vi "Measurement Logic.vi"() -> ()   [LabVIEW 2021, in "Arbitrary Mode_PMIC.lvlib"]
uses:
  Arbitrary Mode_PMIC.lvlib
  <vilib>/Plug-In SDKs/Measurements/Measure Call Context/Measure Call Context.lvclass
  Measurement Results.ctl
  Measurement Configuration.ctl
  <instrlib>/niDCPower/nidcpower.llb/niDCPower Source Mode.ctl
  <instrlib>/niDCPower/nidcpower.llb/niDCPower Wait For Event - Event.ctl
  <instrlib>/niScope/Controls/niScope trigger slope.ctl
  <instrlib>/niDCPower/nidcpower.llb/niDCPower Output Function.ctl
  <instrlib>/niDCPower/nidcpower.llb/niDCPower Aperture Time Units.ctl
  <instrlib>/niDCPower/nidcpower.llb/niDCPower Get Channel Name From String.vi
  <instrlib>/niScope/Utility/niScope Get Channel Name From String.vi
  <instrlib>/niScope/Configure/Trigger/niScope Configure Trigger Digital.vi
  <instrlib>/niDCPower/nidcpower.llb/niDCPower Configure Digital Edge Measure Trigger With Channels.vi
  <instrlib>/niDCPower/nidcpower.llb/niDCPower Configure Digital Edge Source Trigger With Channels.vi
  <instrlib>/niScope/Acquire/Fetch/niScope Fetch WDT.vi
panel:
  in  "measurement configuration":T1={"Source maximum power"=300.0, "Source sample rate"=1800000.0, "Source current limit"=0.25, "Source resource name"="", "Source voltage pole-zero ratio"=2.0, "Source voltage compensation frequency"=3530.0, "Source voltage gain bandwidth"=2000.0, "Source transient response"=1042, "Source set-up voltage"=0.0, "Trapezoid signal enable/disable"=TRUE, "Trapezoid voltage delay t2"=0.005, "Trapezoid voltage delay t1"=0.005, "Trapezoid voltatge pulse duration"=0.005, "Trapezoid voltage rising slew rate"=24.0, "Trapezoid voltage falling slew rate"=24.0, "Trapezoid voltage set point 2(V2)"=20.0, "Trapezoid voltage set point 1(V1)"=7.0, "Ramp signal enable/disable"=FALSE, "Ramp voltage V1 time"=0.005, "Ramp voltatge V2 time"=0.005, "Ramp voltage ramp rate"=6550.0, "Ramp voltage set point 2(V2)"=20.0, "Ramp voltage set point 1(V1)"=7.0, "Source signal logging"=[], "Source signal loop count"=1, "Source sense"=1009, "Load enable/disable"=FALSE, "Load resource name"="", "Load sense"=1009, "Load voltage limit range"=4.0, "Load current level range"=4.0, "Load current level"=0.03, "Load transient response"=1042, "Load current gain bandwidth"=14000.0, "Load current compensation frequency"=180000.0, "Load current pole-zero ratio"=0.3, "Scope enable/disable"=FALSE, "Scope resource name"="", "Scope output channel name"="0", "Scope sample rate"=1800000.0, "Scope probe attenuation"=1.0, "Scope vertical range"=10.0, "Scope vertical coupling"=enum."DC", "Setup time"=1.0} {"Scope vertical range" format="%.2f"; "Scope probe attenuation" format="%.1f"; "Scope sample rate" step=1000000.0 format="%#.2g"; "Load transient response" items=["Slow"=1041, "Normal"=1038, "Fast"=1039, "Custom"=1042]; "Load sense" items=["Local"=1008, "Remote"=1009]; "Source sense" items=["Local"=1008, "Remote"=1009]; "Source signal logging" items=["Trapezoid", "Ramp"]; "Ramp voltage V1 time" format="%#_8g"; "Trapezoid voltage rising slew rate" format="%#_6p"; "Trapezoid voltatge pulse duration" format="%#_6p"; "Source transient response" items=["Slow"=1041, "Normal"=1038, "Fast"=1039, "Custom"=1042]}
  out "measurement results":T2
  out "measure call context out":refnum<class "Measure Call Context.lvclass">
  in  "measure call context in":refnum<class "Measure Call Context.lvclass">
  out "error out":errorcluster
  in  "error in":errorcluster
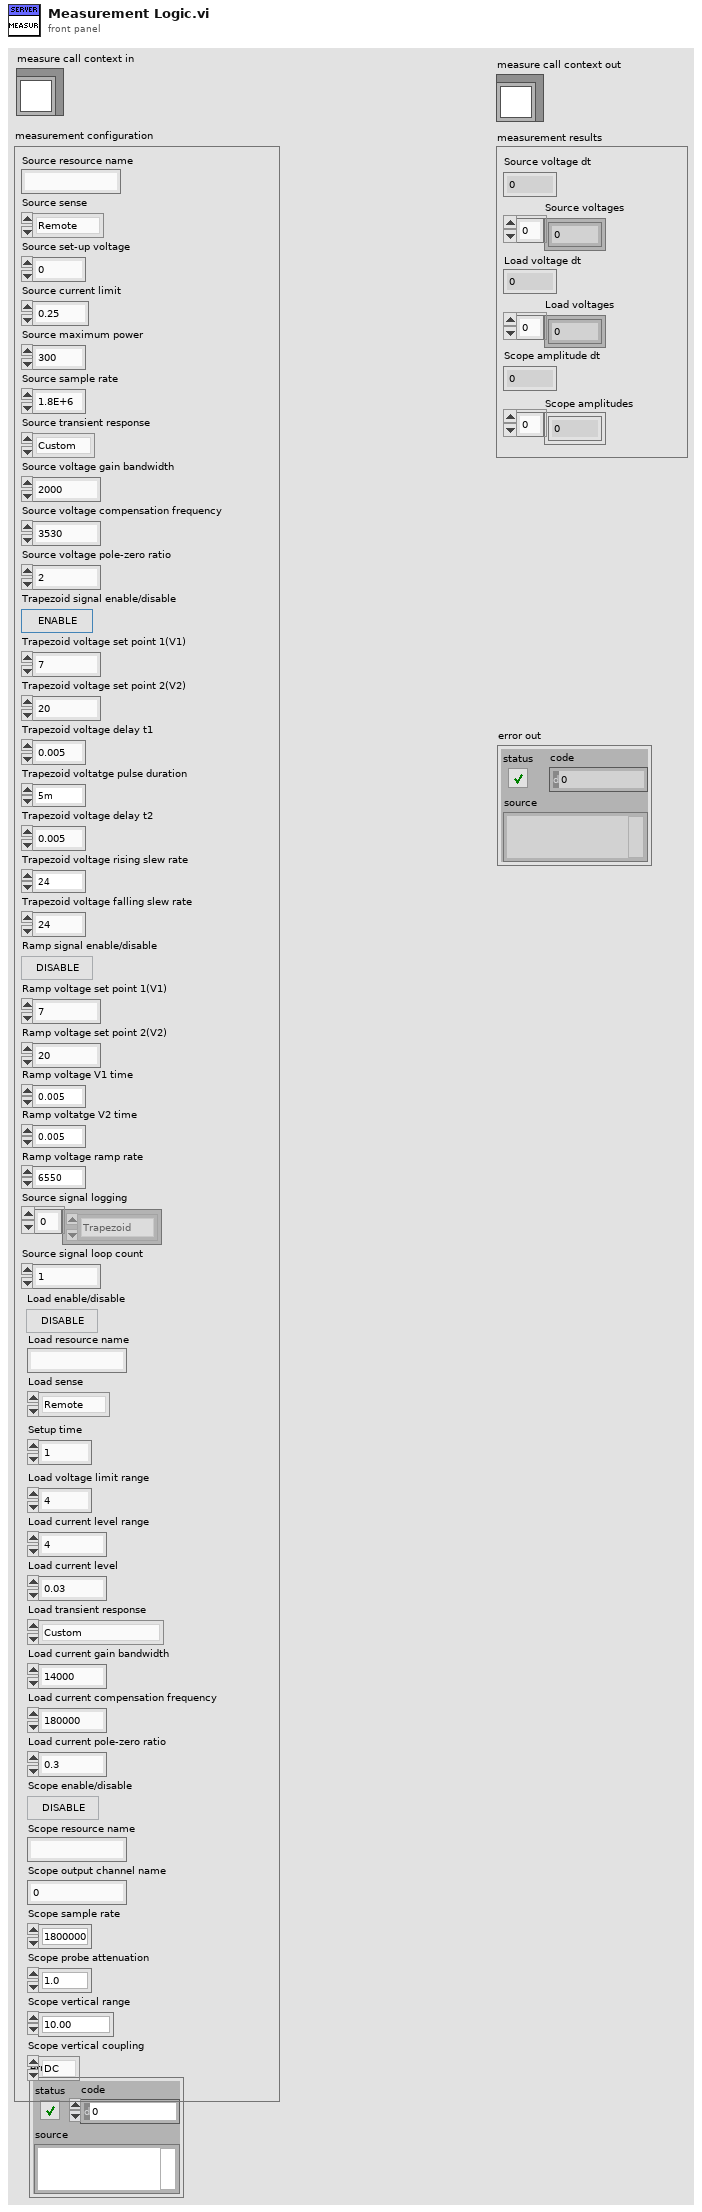
[diagram p1: front panel]
types:
  T1 = typedef "Arbitrary Mode_PMIC.lvlib/Measurement Configuration.ctl" = cluster{"Source maximum power":dbl, "Source sample rate":dbl, "Source current limit":dbl, "Source resource name":string, "Source voltage pole-zero ratio":dbl, "Source voltage compensation frequency":dbl, "Source voltage gain bandwidth":dbl, "Source transient response":i32, "Source set-up voltage":dbl, "Trapezoid signal enable/disable":bool, "Trapezoid voltage delay t2":dbl, "Trapezoid voltage delay t1":dbl, "Trapezoid voltatge pulse duration":dbl, "Trapezoid voltage rising slew rate":dbl, "Trapezoid voltage falling slew rate":dbl, "Trapezoid voltage set point 2(V2)":dbl, "Trapezoid voltage set point 1(V1)":dbl, "Ramp signal enable/disable":bool, "Ramp voltage V1 time":dbl, "Ramp voltatge V2 time":dbl, "Ramp voltage ramp rate":dbl, "Ramp voltage set point 2(V2)":dbl, "Ramp voltage set point 1(V1)":dbl, "Source signal logging":u32[], "Source signal loop count":i64, "Source sense":i32, "Load enable/disable":bool, "Load resource name":string, "Load sense":i32, "Load voltage limit range":dbl, "Load current level range":dbl, "Load current level":dbl, "Load transient response":i32, "Load current gain bandwidth":dbl, "Load current compensation frequency":dbl, "Load current pole-zero ratio":dbl, "Scope enable/disable":bool, "Scope resource name":string, "Scope output channel name":string, "Scope sample rate":dbl, "Scope probe attenuation":dbl, "Scope vertical range":dbl, "Scope vertical coupling":enum32{"AC", "DC"}, "Setup time":dbl}
  T2 = typedef "Arbitrary Mode_PMIC.lvlib/Measurement Results.ctl" = cluster{"Source voltage dt":dbl, "Source voltages":dbl[], "Load voltage dt":dbl, "Load voltages":dbl[], "Scope amplitudes":dbl[], "Scope amplitude dt":dbl}
  T3 = cluster{"Source out":refnum<k15>, "Source channel name":string, "Load out":refnum<k15>, "Load channel name":string, "Scope out":refnum<k15>, "Scope channel name":string, "Source terminal name":string, "Start source terminal name":string, "Measure load and scope terminal name":string, "Measure record length smu":i32, "Aperture time":dbl, "Measure record length scope":i32, "Measurement Results":T2}
  T4 = typedef "niDCPower Wait For Event - Event.ctl" = i32
  T5 = typedef "niDCPower Source Mode.ctl" = i32
  T6 = typedef "niScope trigger slope.ctl" = i32
  T7 = typedef "niDCPower Aperture Time Units.ctl" = i32
  T8 = typedef "niDCPower Output Function.ctl" = i32
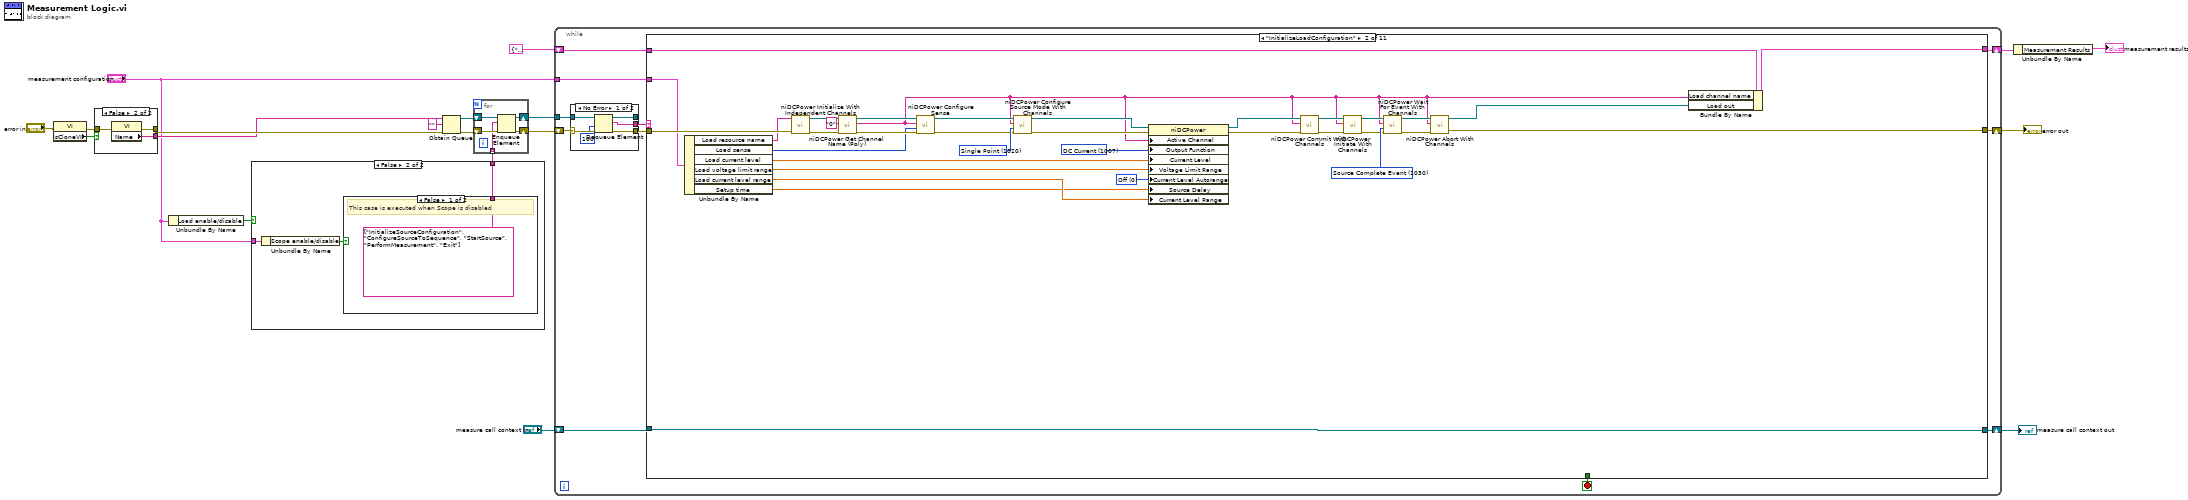
[diagram p0: block diagram]
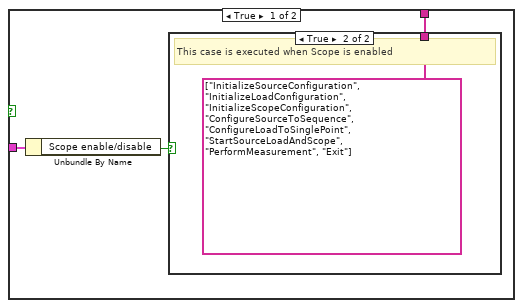
[diagram p2: hidden frame]
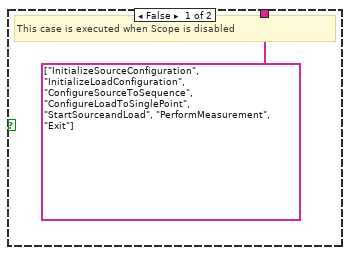
[diagram p3: hidden frame]
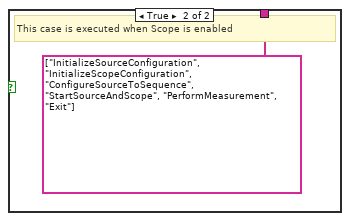
[diagram p4: hidden frame]
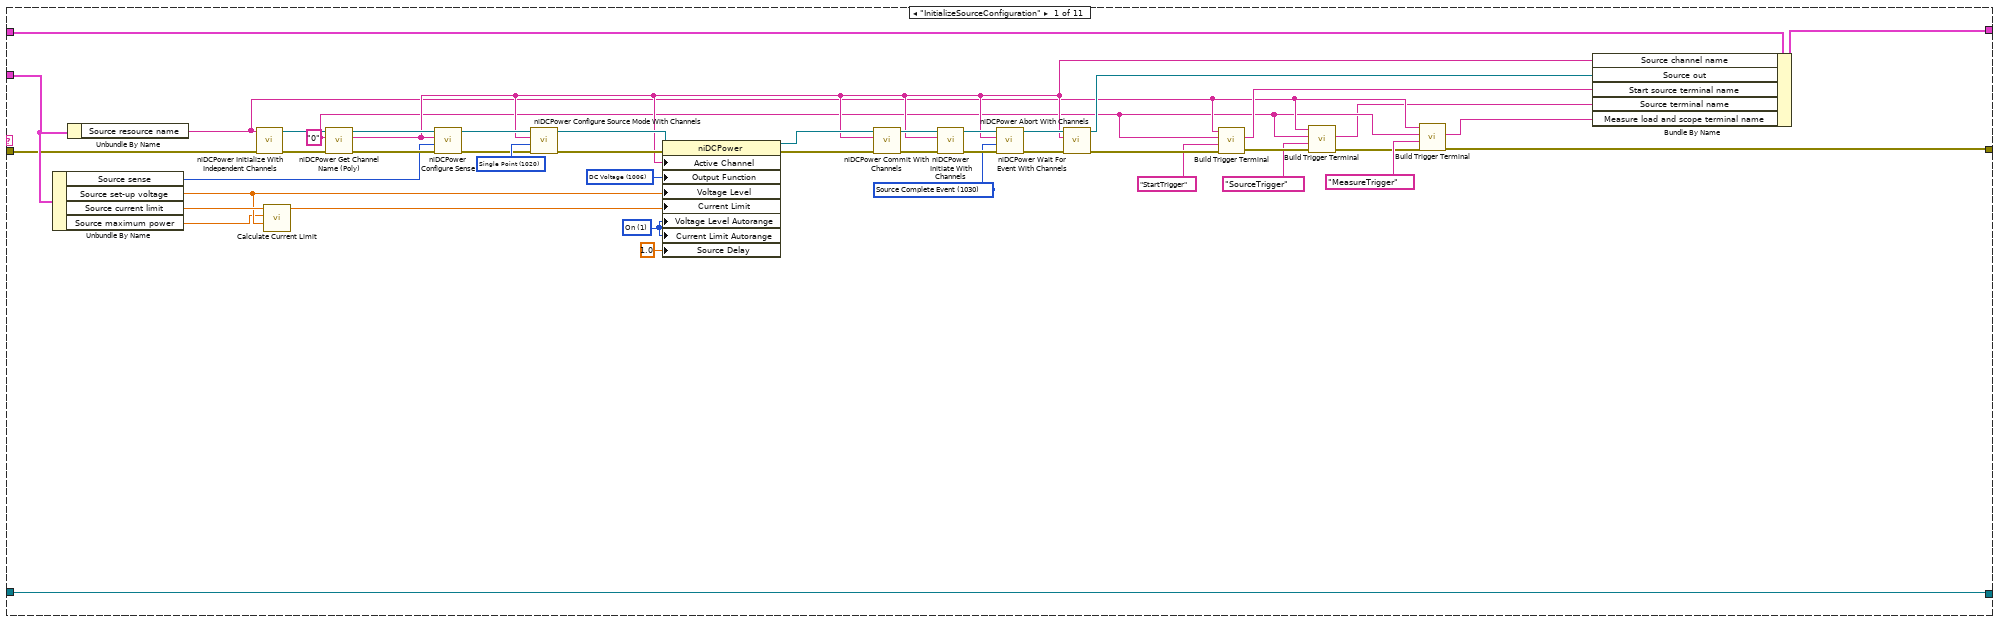
[diagram p5: hidden frame]
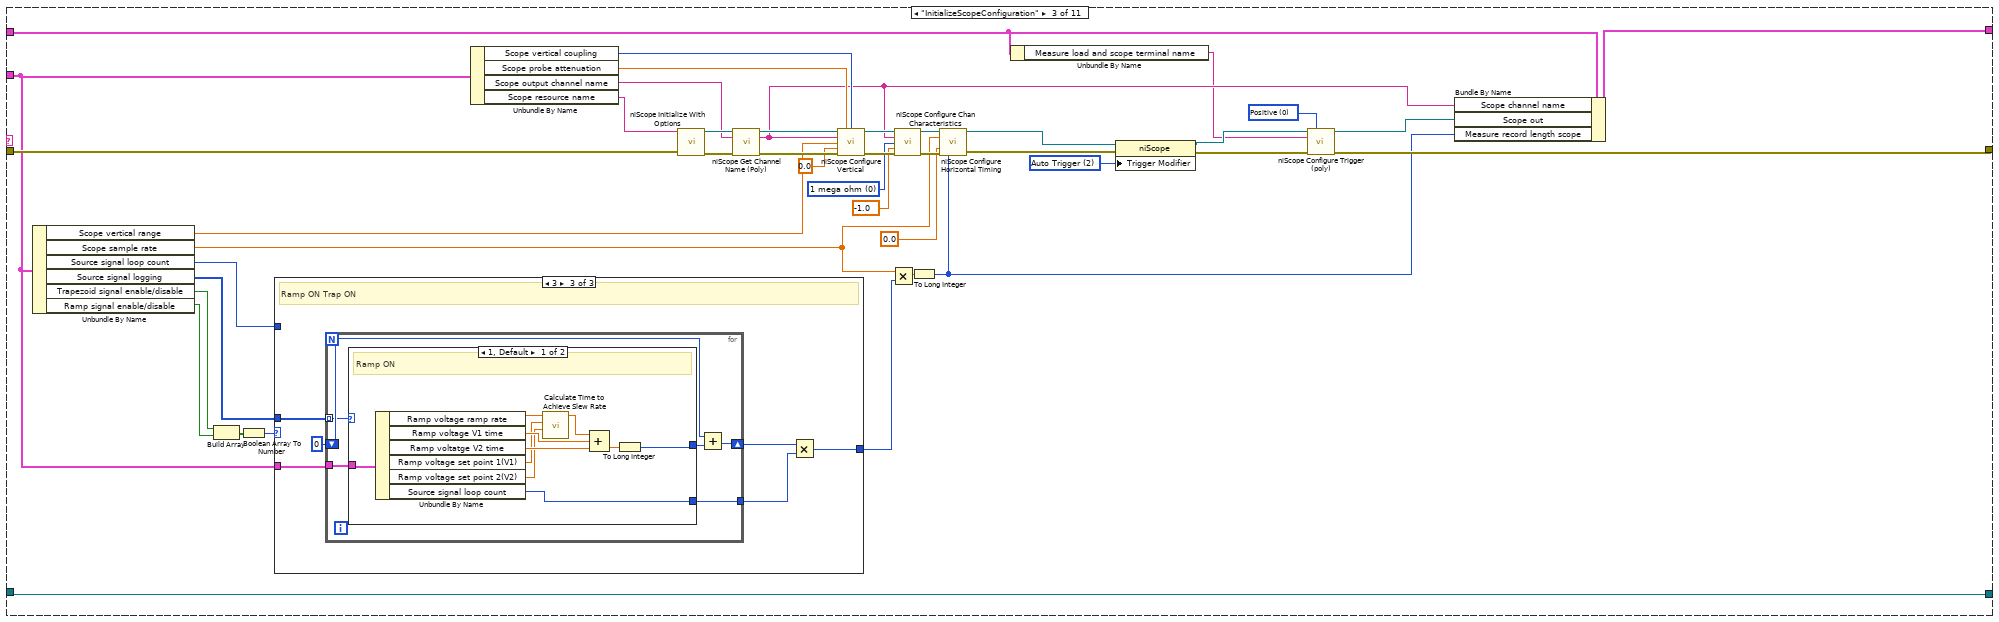
[diagram p6: hidden frame]
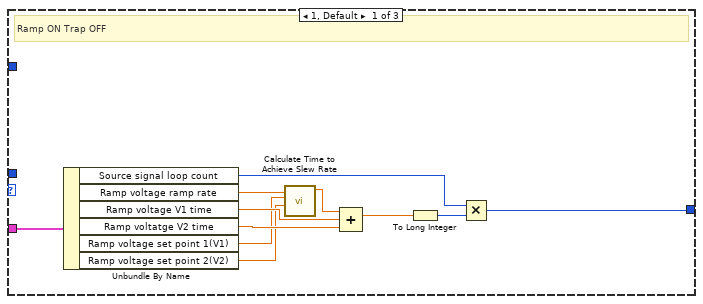
[diagram p7: hidden frame]
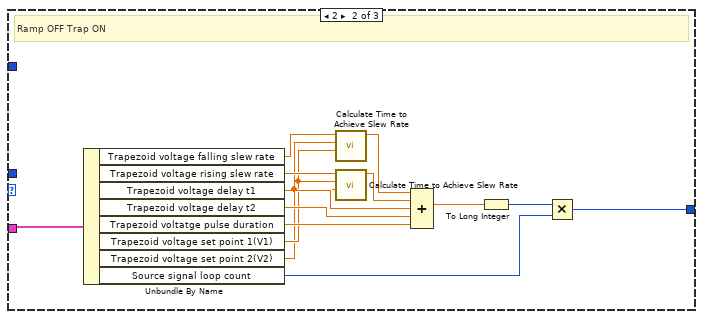
[diagram p8: hidden frame]
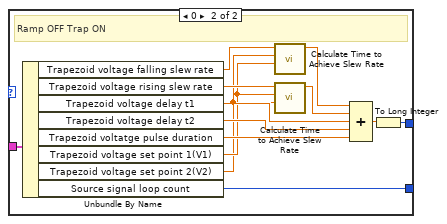
[diagram p9: hidden frame]
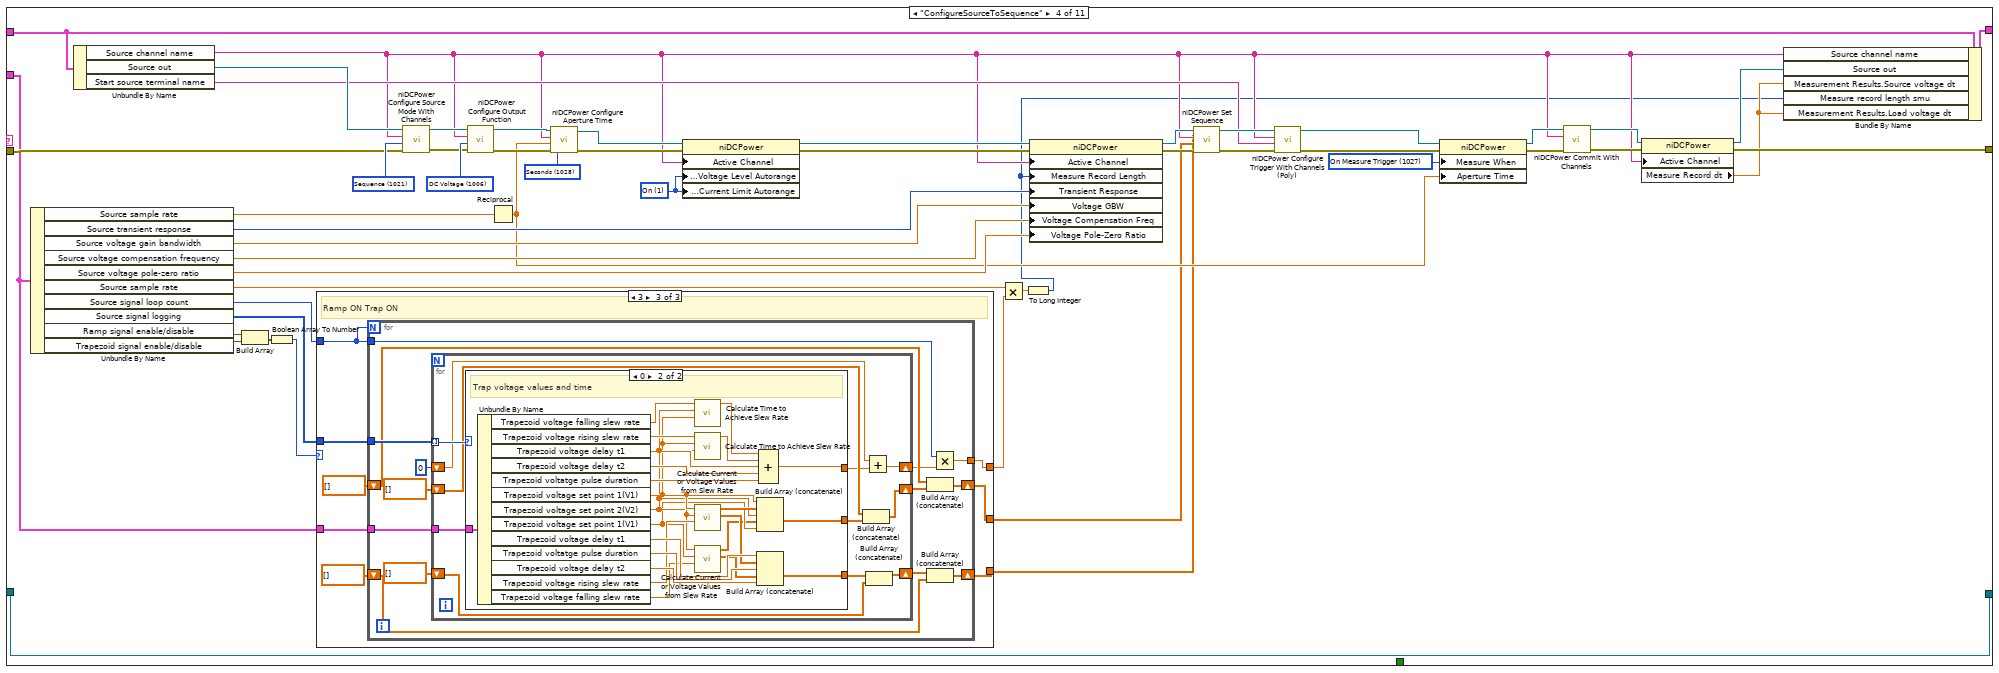
[diagram p10: hidden frame]
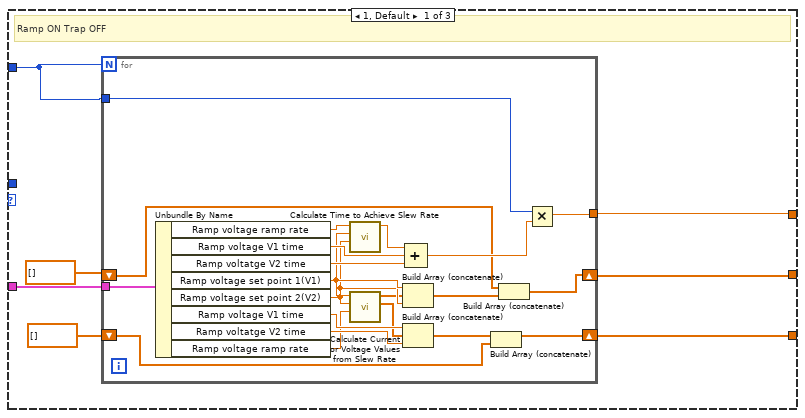
[diagram p11: hidden frame]
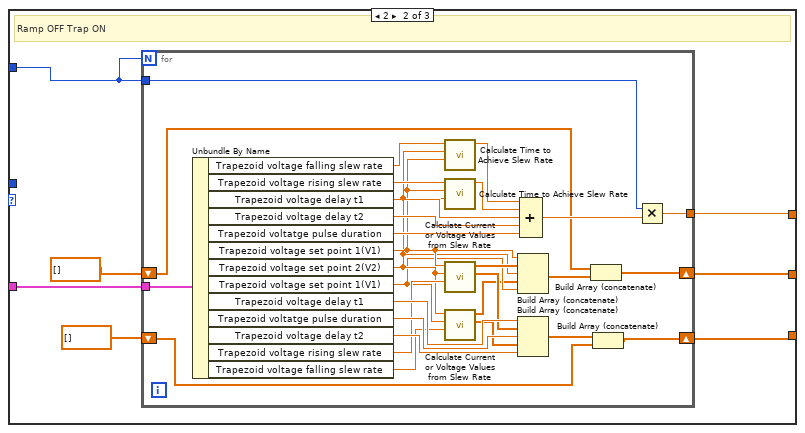
[diagram p12: hidden frame]
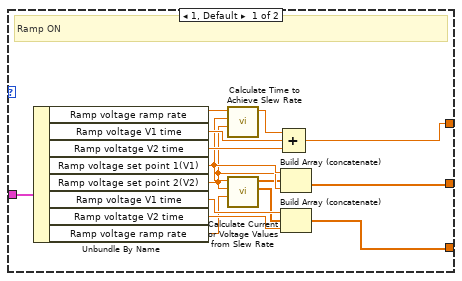
[diagram p13: hidden frame]
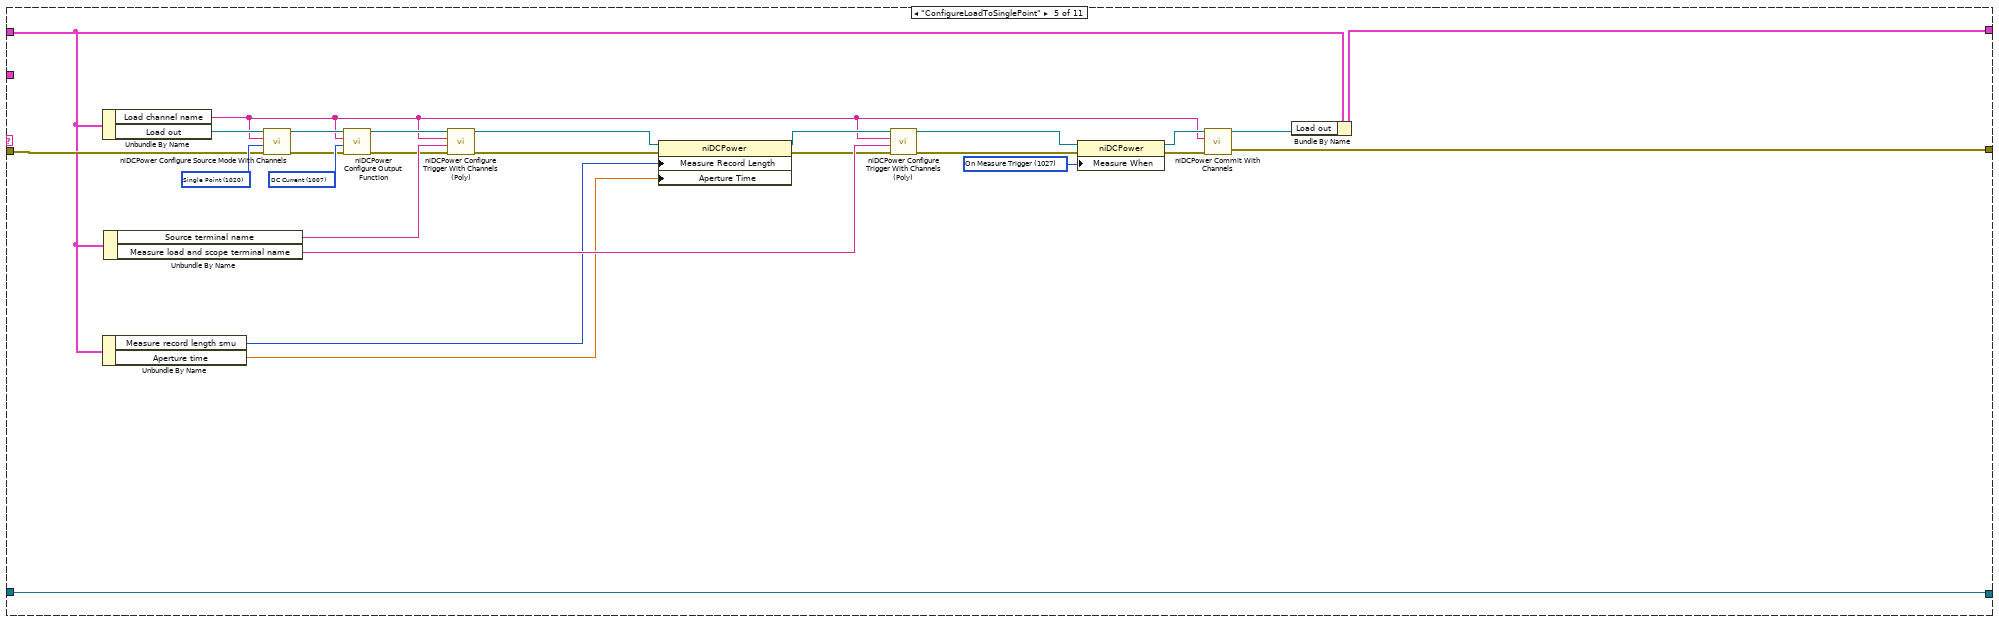
[diagram p14: hidden frame]
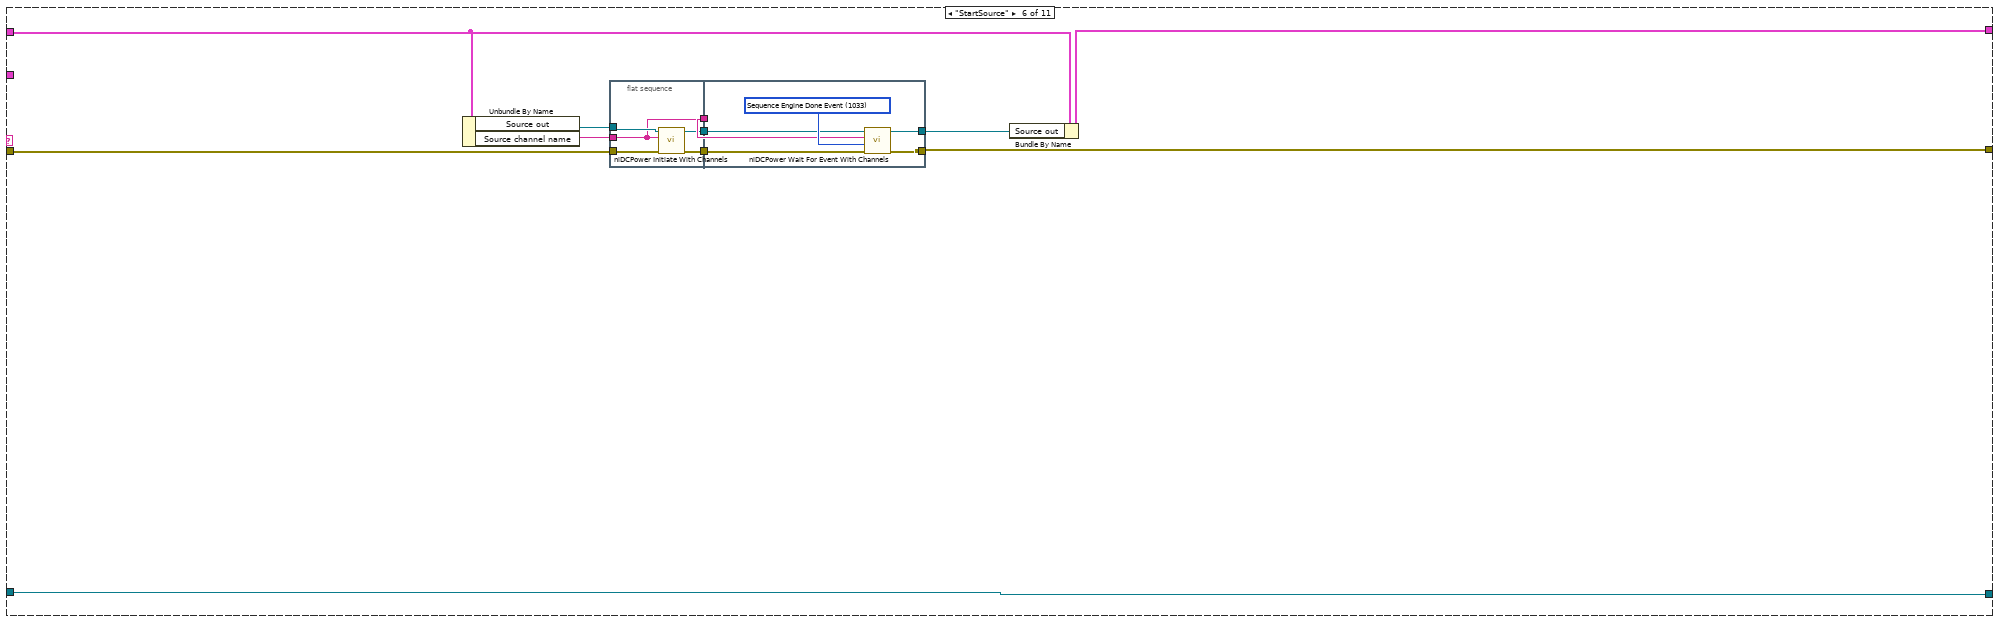
[diagram p15: hidden frame]
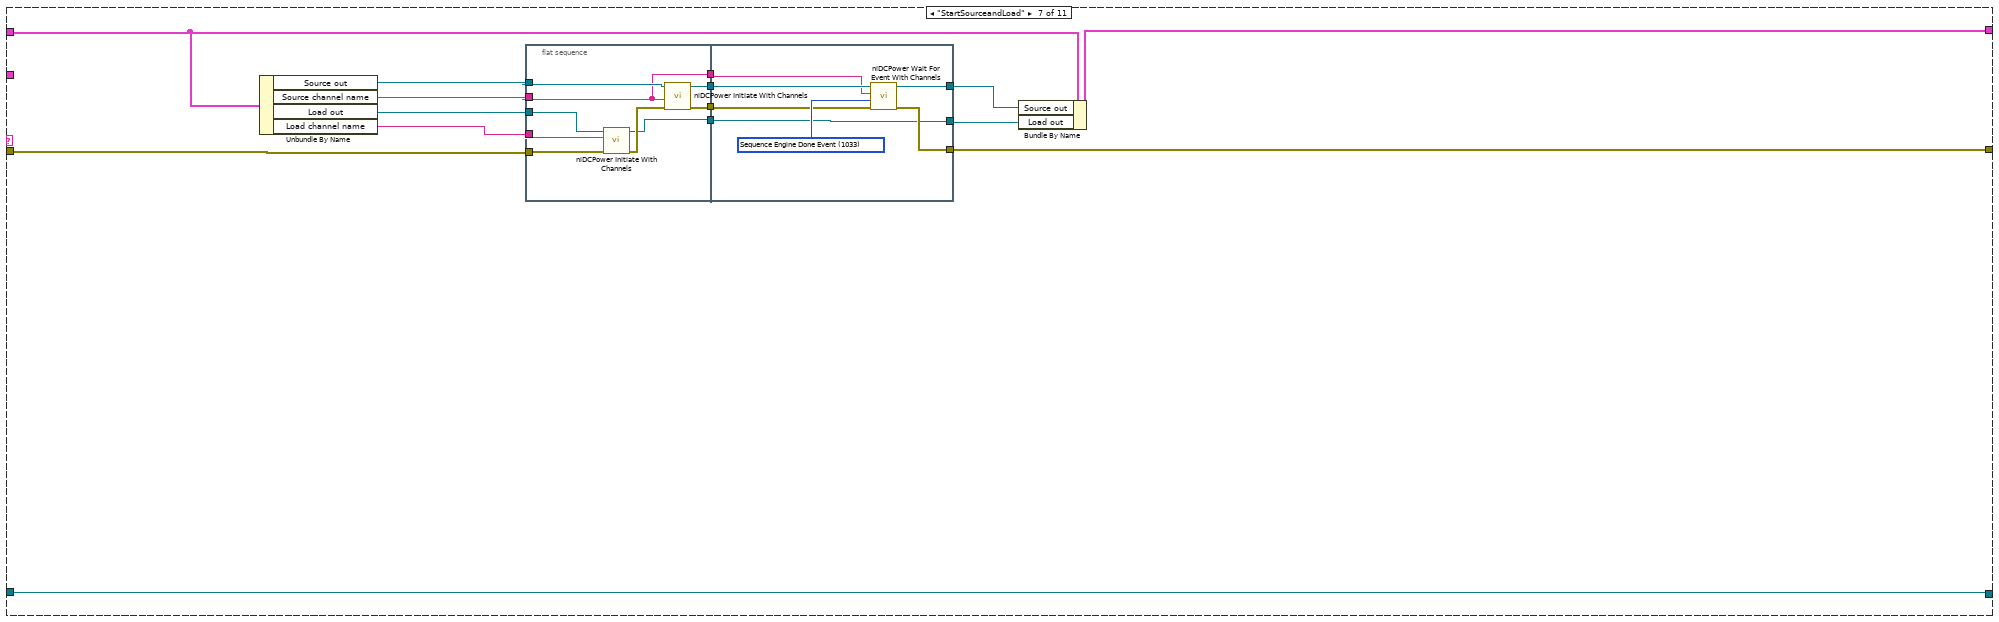
[diagram p16: hidden frame]
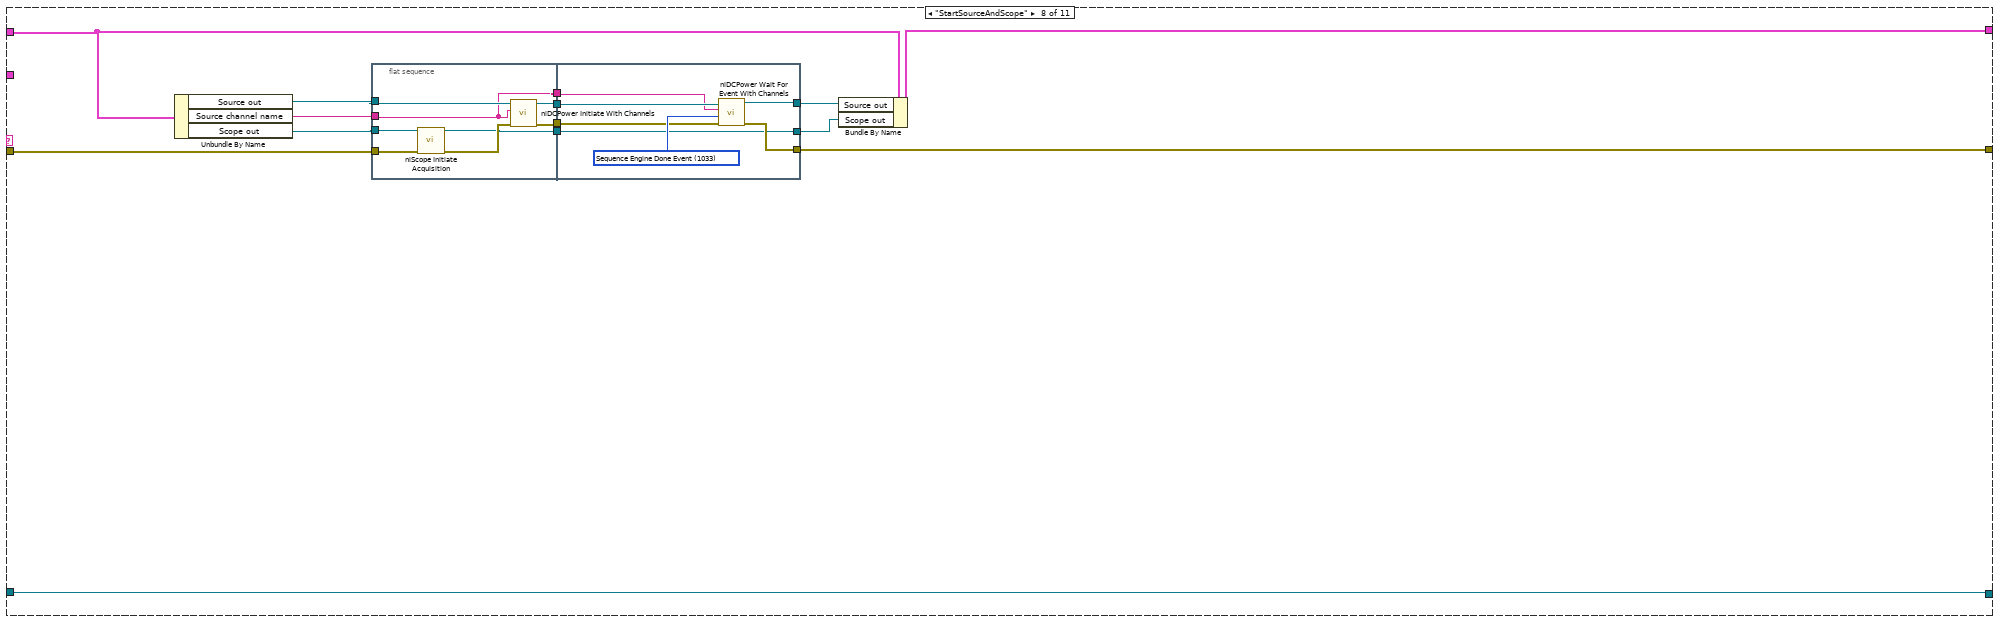
[diagram p17: hidden frame]
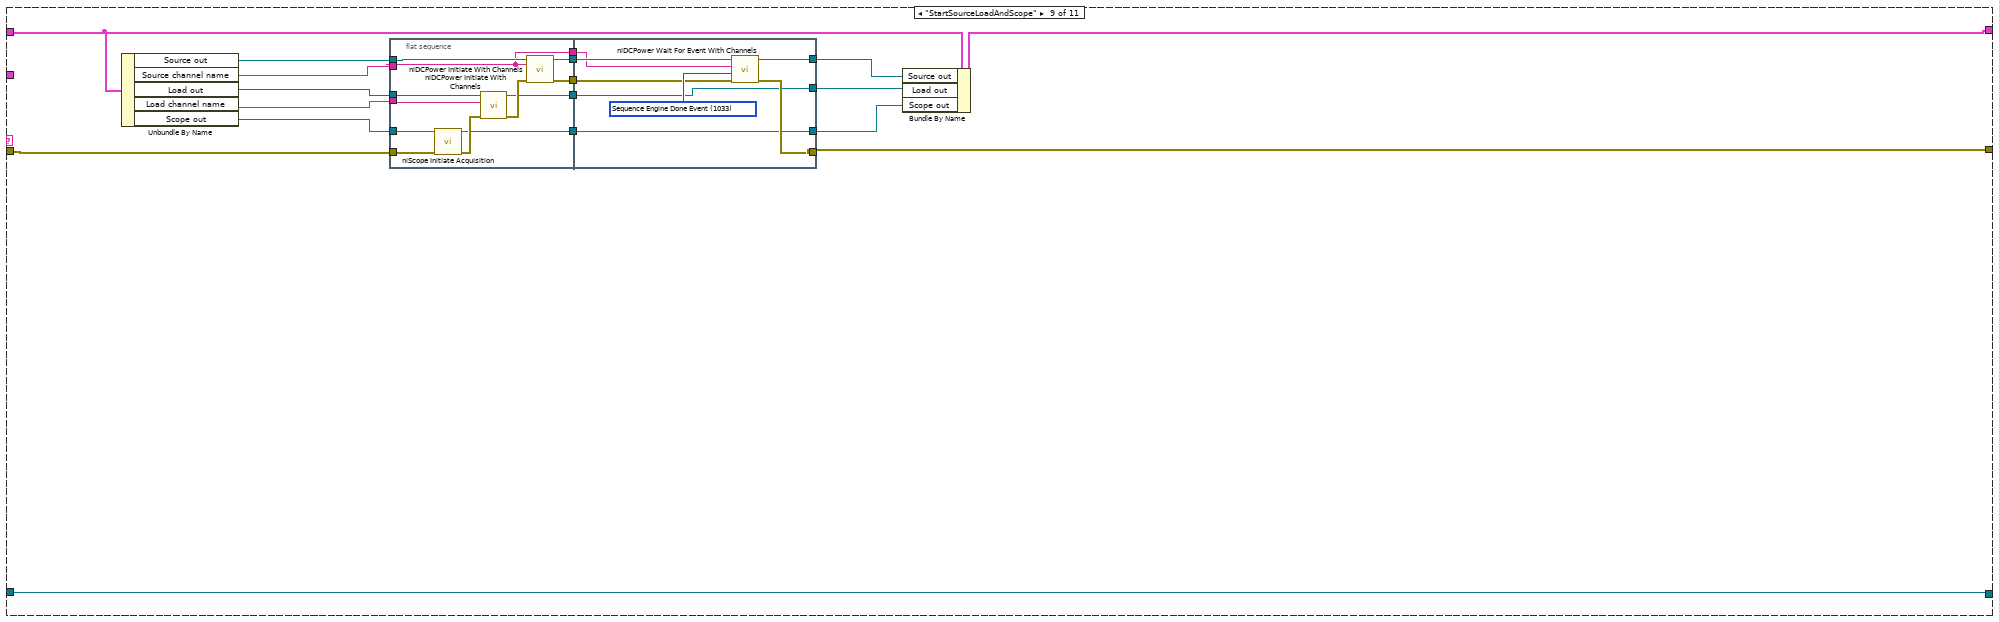
[diagram p18: hidden frame]
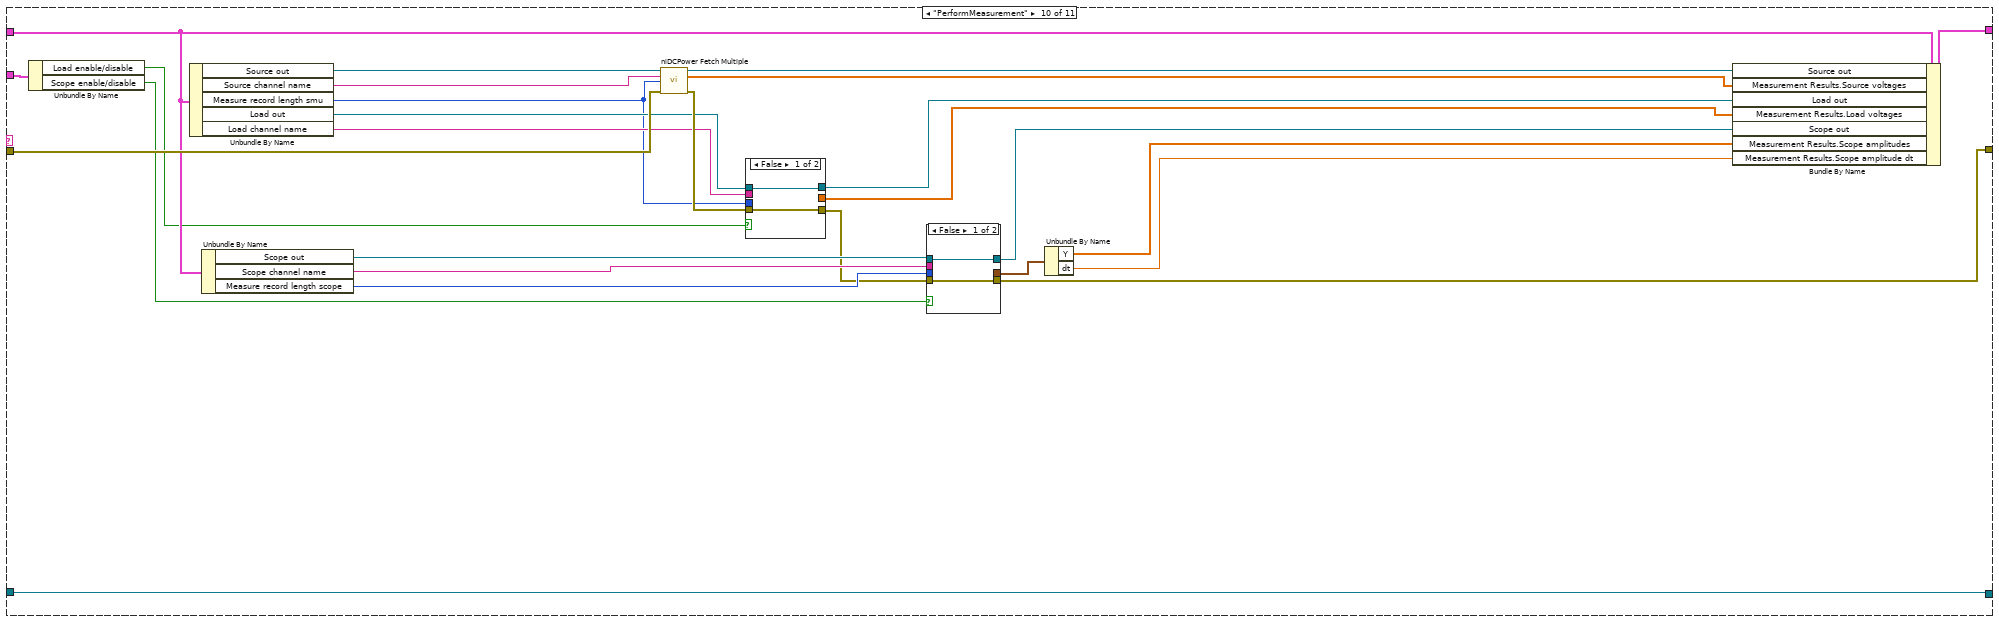
[diagram p19: hidden frame]
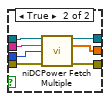
[diagram p20: hidden frame]
diagram:
  n1 = property class="VI"(error in="error in") -> (error out=w18:errorcluster, "IsCloneVI"=w19:bool)  [unwired: 1 in, 1 out]
  n2 = case shown="False" w19 {
    tunnel: [w22 w25] -> w17
    tunnel: [w21 w24] -> w16
    tunnel: w18 -> [w20 w23]
    frame True {
      n3 = property class="VI"(error in=w20) -> (error out=w22:errorcluster, "Clone Name"=w21:string)  [unwired: 1 in, 1 out]
    }
    frame False {
      n4 = property class="VI"(error in=w23) -> (error out=w25:errorcluster, "Name"=w24:string)  [unwired: 1 in, 1 out]
    }
  }
  n5 = Unbundle By Name("measurement configuration") -> ("Load enable/disable"=w4:bool)
  n6 = case shown="False" w4 {
    tunnel: [w26 w33] -> w12
    tunnel: "measurement configuration" -> [w27 w31]
    frame True {
      n7 = Unbundle By Name(w27) -> ("Scope enable/disable"=w28:bool)
      n8 = case shown="True" w28 {
        tunnel: [string[] ["InitializeSourceConfiguration", "InitializeLoadConfiguration", "ConfigureSourceToSequence", "ConfigureLoadToSinglePoint", "StartSourceandLoad", "PerformMeasurement", "Exit"] ("Step sequence") string[] ["InitializeSourceConfiguration", "InitializeLoadConfiguration", "InitializeScopeConfiguration", "ConfigureSourceToSequence", "ConfigureLoadToSinglePoint", "StartSourceLoadAndScope", "PerformMeasurement", "Exit"] ("Step sequence")] -> w26
        frame False {
          # "This case is executed when Scope is disabled"
        }
        frame True {
          # "This case is executed when Scope is enabled"
        }
      }
    }
    frame False {
      n9 = Unbundle By Name(w31) -> ("Scope enable/disable"=w32:bool)
      n10 = case shown="False" w32 {
        tunnel: [string[] ["InitializeSourceConfiguration", "ConfigureSourceToSequence", "StartSource", "PerformMeasurement", "Exit"] ("Step sequence") string[] ["InitializeSourceConfiguration", "InitializeScopeConfiguration", "ConfigureSourceToSequence", "StartSourceAndScope", "PerformMeasurement", "Exit"] ("Step sequence")] -> w33
        frame False {
          # "This case is executed when Scope is disabled"
        }
        frame True {
          # "This case is executed when Scope is enabled"
        }
      }
    }
  }
  n11 = Obtain Queue(name (unnamed)=w16, element data type="", error in (no error)=w17) -> (queue out=w14:refnum<queue>, error out=w15:errorcluster)  [unwired: 2 in, 1 out]
  n12 = for {
    shift-right: [w38] -> w11
    shift-left: w14 -> [w40]
    shift-right: [w37] -> w10
    shift-left: w15 -> [w39]
    tunnel: w12 -> [w36] mode=indexing
    n13 = Enqueue Element(queue=w40, element=w36, error in (no error)=w39) -> (queue out=w38:refnum<queue>, error out=w37:errorcluster)  [unwired: 1 in, 1 out]
  }
  n14 = while {
    tunnel: w11 -> [w51]
    shift-right: [w44] -> w5
    shift-left: w10 -> [w50]
    tunnel: "measurement configuration" -> [w48]
    shift-right: [w46] -> w3
    shift-left: T3 {"Source out"="", "Source channel name"="", "Load out"="", "Load channel name"="", "Scope out"="", "Scope channel name"="", "Source terminal name"="", "Start source terminal name"="", "Measure load and scope terminal name"="", "Measure record length smu"=0, "Aperture time"=0.0, "Measure record length scope"=0, "Measurement Results"={"Source voltage dt"=0.0, "Source voltages"=[], "Load voltage dt"=0.0, "Load voltages"=[], "Scope amplitudes"=[], "Scope amplitude dt"=0.0}} -> [w47]
    shift-right: [w42] -> w6
    shift-left: "measure call context in" -> [w41]
    stop <- w43 stop-if-true
    n15 = case shown="No Error" w50 {
      selector: w50 -> [w643 w647]
      tunnel: w51 -> [w645 w646]
      tunnel: [w644 "Exit" ("t")] -> w49
      tunnel: [w642 w647] -> w45
      tunnel: [w640 w646] -> _
      frame No Error {
        n16 = Dequeue Element(queue=w645, timeout in ms (-1)=100, error in (no error)=w643) -> (queue out=w640:refnum<queue>, element=w644:string, error out=w642:errorcluster)  [unwired: 1 out]
      }
      frame Error {
      }
    }
    n17 = case shown="\"InitializeLoadConfiguration\"" w49 {
      tunnel: w48 -> [w74 w103 w142 w248 _ _ _ _ _ w573 w624]
      tunnel: w47 -> [w73 w100 w146 w259 w423 w452 w472 w508 w532 w592 w625]
      tunnel: [w72 w101 w173 w285 w422 w451 w471 w503 w531 w591 w625] -> w46
      tunnel: w45 -> [w71 w104 w149 w257 w424 w453 w473 w507 w533 w593 w628]
      tunnel: [w57 w102 w144 w249 w421 w450 w470 w504 w530 w590 w627] -> w44
      tunnel: [_ _ _ _ _ _ _ _ _ _ TRUE] -> w43
      tunnel: [w69 w131 w143 w254 w447 w449 w484 w502 w547 w582 w618] -> w42
      tunnel: w41 -> [w69 w131 w143 w254 w447 w449 w484 w502 w547 w582 w618]
      frame "InitializeSourceConfiguration" {
        w55 = "0" ("index")
        w80 = 1 items=["Off", "On"] ("Source:DC Voltage:Voltage Level Autorange")
        w81 = T4 1030 items=["Source Complete Event"=1030, "Measure Complete Event"=1031, "Sequence Iteration Complete Event"=1032, "Sequence Engine Done Event"=1033, "Pulse Complete Event"=1051, "Ready For Pulse Trigger Event"=1052] ("event")
        w92 = T5 1020 items=["Single Point"=1020, "Sequence"=1021] ("source mode")
        w87 = 1006 items=["DC Voltage"=1006, "DC Current"=1007, "Pulse Voltage"=1049, "Pulse Current"=1050] ("Source:Output Function")
        n18 = Unbundle By Name(w74) -> ("Source sense"=w52:i32, "Source set-up voltage"=w67:dbl, "Source current limit"=w68:dbl, "Source maximum power"=w66:dbl)
        n19 = Unbundle By Name(w74) -> ("Source resource name"=w56:string)
        n20 = call <instrlib>:"niDCPower Initialize With Independent Channels.vi"("error in (no error)"=w71, "resource name"=w56) -> ("error out"=w78:errorcluster, "instrument handle out"=w82:refnum<k15>)  [unwired: 8 in]
        n21 = call "Calculate Current Limit.vi"("Voltage value"=w67, "Maximum power"=w66, "Current limit in"=w68) -> ("Current limit out"=w65:dbl)  [unwired: 8 in]
        n22 = call-poly <instrlib>:"niDCPower Get Channel Name (Poly).vi"("error in (no error)"=w78, "index"=w55, "instrument handle"=w82) -> ("error out"=w77:errorcluster, "name"=w76:string, "instrument handle out"=w79:refnum<k15>)  [unwired: 6 in]
        n23 = call <instrlib>:"niDCPower Configure Sense.vi"("error in (no error)"=w77, "sense"=w52, "channel name"=w76, "instrument handle"=w79) -> ("error out"=w90:errorcluster, "instrument handle out"=w88:refnum<k15>)  [unwired: 6 in]
        n24 = call <instrlib>:"niDCPower Configure Source Mode With Channels.vi"("error in (no error)"=w90, "source mode"=w92, "channel name"=w76, "instrument handle"=w88) -> ("error out"=w91:errorcluster, "instrument handle out"=w89:refnum<k15>)  [unwired: 6 in]
        n25 = property class="niDCPower"(reference=w89, error in=w91, "Active Channel"=w76, "Output Function"=w87, "Voltage Level"=w67, "Current Limit"=w65, "Voltage Level Autorange"=w80, "Current Limit Autorange"=w80, "Source Delay"=1.0 ("Source:Advanced:Source Delay")) -> (reference out=w93:refnum<k15>, error out=w94:errorcluster)
        n26 = call <instrlib>:"niDCPower Commit With Channels.vi"("error in (no error)"=w94, "channel name"=w76, "instrument handle"=w93) -> ("error out"=w96:errorcluster, "instrument handle out"=w95:refnum<k15>)  [unwired: 7 in]
        n27 = call <instrlib>:"niDCPower Initiate With Channels.vi"("error in (no error)"=w96, "channel name"=w76, "instrument handle"=w95) -> ("error out"=w83:errorcluster, "instrument handle out"=w84:refnum<k15>)  [unwired: 7 in]
        n28 = call <instrlib>:"niDCPower Wait For Event With Channels.vi"("error in (no error)"=w83, "event"=w81, "channel name"=w76, "instrument handle"=w84) -> ("error out"=w86:errorcluster, "instrument handle out"=w85:refnum<k15>)  [unwired: 6 in]
        n29 = call <instrlib>:"niDCPower Abort With Channels.vi"("error in (no error)"=w86, "channel name"=w76, "instrument handle"=w85) -> ("error out"=w64:errorcluster, "instrument handle out"=w75:refnum<k15>)  [unwired: 7 in]
        n30 = call "Build Trigger Terminal.vi"("error in (no error)"=w64, "Trigger/Event Name"="StartTrigger", "Channel Name"=w55, "Resource Name"=w56) -> ("error out"=w62:errorcluster, "Terminal Name"=w60:string)  [unwired: 6 in]
        n31 = call "Build Trigger Terminal.vi"("error in (no error)"=w62, "Trigger/Event Name"="SourceTrigger", "Channel Name"=w55, "Resource Name"=w56) -> ("error out"=w58:errorcluster, "Terminal Name"=w53:string)  [unwired: 6 in]
        n32 = call "Build Trigger Terminal.vi"("error in (no error)"=w58, "Trigger/Event Name"="MeasureTrigger", "Channel Name"=w55, "Resource Name"=w56) -> ("error out"=w57:errorcluster, "Terminal Name"=w54:string)  [unwired: 6 in]
        n33 = Bundle By Name(cluster=w73, "Source channel name"=w76, "Source out"=w75, "Start source terminal name"=w60, "Source terminal name"=w53, "Measure load and scope terminal name"=w54) -> (w72:T3)
      }
      frame "InitializeLoadConfiguration" {
        w126 = T5 1020 items=["Single Point"=1020, "Sequence"=1021] ("source mode")
        w119 = T4 1030 items=["Source Complete Event"=1030, "Measure Complete Event"=1031, "Sequence Iteration Complete Event"=1032, "Sequence Engine Done Event"=1033, "Pulse Complete Event"=1051, "Ready For Pulse Trigger Event"=1052] ("event")
        w114 = 0 items=["Off", "On"] ("Source:DC Current:Current Level Autorange")
        w115 = 1007 items=["DC Voltage"=1006, "DC Current"=1007, "Pulse Voltage"=1049, "Pulse Current"=1050] ("Source:Output Function")
        n34 = Unbundle By Name(w103) -> ("Load resource name"=w99:string, "Load sense"=w98:i32, "Load current level"=w109:dbl, "Load voltage limit range"=w108:dbl, "Load current level range"=w107:dbl, "Setup time"=w97:dbl)
        n35 = call <instrlib>:"niDCPower Initialize With Independent Channels.vi"("error in (no error)"=w104, "resource name"=w99) -> ("error out"=w112:errorcluster, "instrument handle out"=w116:refnum<k15>)  [unwired: 8 in]
        n36 = call-poly <instrlib>:"niDCPower Get Channel Name (Poly).vi"("error in (no error)"=w112, "index"="0", "instrument handle"=w116) -> ("error out"=w111:errorcluster, "name"=w105:string, "instrument handle out"=w113:refnum<k15>)  [unwired: 6 in]
        n37 = call <instrlib>:"niDCPower Configure Sense.vi"("error in (no error)"=w111, "sense"=w98, "channel name"=w105, "instrument handle"=w113) -> ("error out"=w123:errorcluster, "instrument handle out"=w122:refnum<k15>)  [unwired: 6 in]
        n38 = call <instrlib>:"niDCPower Configure Source Mode With Channels.vi"("error in (no error)"=w123, "source mode"=w126, "channel name"=w105, "instrument handle"=w122) -> ("error out"=w125:errorcluster, "instrument handle out"=w124:refnum<k15>)  [unwired: 6 in]
        n39 = property class="niDCPower"(reference=w124, error in=w125, "Active Channel"=w105, "Output Function"=w115, "Current Level"=w109, "Voltage Limit Range"=w108, "Current Level Autorange"=w114, "Source Delay"=w97, "Current Level Range"=w107) -> (reference out=w127:refnum<k15>, error out=w128:errorcluster)
        n40 = call <instrlib>:"niDCPower Commit With Channels.vi"("error in (no error)"=w128, "channel name"=w105, "instrument handle"=w127) -> ("error out"=w129:errorcluster, "instrument handle out"=w130:refnum<k15>)  [unwired: 7 in]
        n41 = call <instrlib>:"niDCPower Initiate With Channels.vi"("error in (no error)"=w129, "channel name"=w105, "instrument handle"=w130) -> ("error out"=w117:errorcluster, "instrument handle out"=w118:refnum<k15>)  [unwired: 7 in]
        n42 = call <instrlib>:"niDCPower Wait For Event With Channels.vi"("error in (no error)"=w117, "event"=w119, "channel name"=w105, "instrument handle"=w118) -> ("error out"=w121:errorcluster, "instrument handle out"=w120:refnum<k15>)  [unwired: 6 in]
        n43 = call <instrlib>:"niDCPower Abort With Channels.vi"("error in (no error)"=w121, "channel name"=w105, "instrument handle"=w120) -> ("error out"=w102:errorcluster, "instrument handle out"=w110:refnum<k15>)  [unwired: 7 in]
        n44 = Bundle By Name(cluster=w100, "Load channel name"=w105, "Load out"=w110) -> (w101:T3)
      }
      frame "InitializeScopeConfiguration" {
        w161 = 2 items=["None"=1, "Auto Trigger"=2] ("Trigger Modifier")
        w153 = u32 0 items=["1 mega ohm"=0, "50 ohms"=2] ("Input Impedance")
        w158 = T6 0 items=["Positive", "Negative"] ("trigger slope")
        n45 = Unbundle By Name(w142) -> ("Scope vertical range"=w152:dbl, "Scope sample rate"=w135:dbl, "Source signal loop count"=w132:i64, "Source signal logging"=w137:u32[], "Trapezoid signal enable/disable"=w140:bool, "Ramp signal enable/disable"=w139:bool)
        n46 = Build Array(w140, w139) -> (w141:bool[])
        n47 = Boolean Array To Number(Boolean array=w141) -> (number=w138:u32)
        n48 = case shown="3" w138 {
          tunnel: [w175 w185 w201] -> w136
          tunnel: w142 -> [w178 w189 w204]
          tunnel: w137 -> [_ _ w203]
          tunnel: w132 -> [_ _ _]
          frame 1, Default {
            # "Ramp ON Trap OFF"
            n49 = Unbundle By Name(w178) -> ("Source signal loop count"=w174:i64, "Ramp voltage ramp rate"=w180:dbl, "Ramp voltage V1 time"=w183:dbl, "Ramp voltatge V2 time"=w184:dbl, "Ramp voltage set point 1(V1)"=w182:dbl, "Ramp voltage set point 2(V2)"=w181:dbl)
            n50 = call "Calculate Time to Achieve Slew Rate.vi"("Current/voltage set point 2"=w181, "Current/voltage set point 1"=w182, "Current/voltage slew rate"=w180) -> ("Calculated time"=w179:dbl)  [unwired: 8 in]
            n51 = Compound Arithmetic op=ADD(w179, w183, w184) -> (w177:dbl)
            n52 = To Long Integer(number=w177) -> (32bit integer=w176:i32)
            n53 = Multiply(x=w174, y=w176) -> (x*y=w175:i64)
          }
          frame 2 {
            # "Ramp OFF Trap ON"
            n54 = Unbundle By Name(w189) -> ("Trapezoid voltage falling slew rate"=w195:dbl, "Trapezoid voltage rising slew rate"=w193:dbl, "Trapezoid voltage delay t1"=w198:dbl, "Trapezoid voltage delay t2"=w196:dbl, "Trapezoid voltatge pulse duration"=w197:dbl, "Trapezoid voltage set point 1(V1)"=w191:dbl, "Trapezoid voltage set point 2(V2)"=w190:dbl, "Source signal loop count"=w186:i64)
            n55 = call "Calculate Time to Achieve Slew Rate.vi"("Current/voltage set point 2"=w191, "Current/voltage set point 1"=w190, "Current/voltage slew rate"=w195) -> ("Calculated time"=w194:dbl)  [unwired: 8 in]
            n56 = call "Calculate Time to Achieve Slew Rate.vi"("Current/voltage set point 2"=w190, "Current/voltage set point 1"=w191, "Current/voltage slew rate"=w193) -> ("Calculated time"=w192:dbl)  [unwired: 8 in]
            n57 = Compound Arithmetic op=ADD(w194, w192, w198, w196, w197) -> (w188:dbl)
            n58 = To Long Integer(number=w188) -> (32bit integer=w187:i32)
            n59 = Multiply(x=w187, y=w186) -> (x*y=w185:i64)
          }
          frame 3 {
            # "Ramp ON Trap ON"
            n60 = for {
              shift-right: [w210] -> w200
              shift-left: 0 -> [w209]
              tunnel: w204 -> [w208]
              tunnel: w203 -> [w206] mode=indexing
              tunnel: [w205] -> w199
              n61 = case shown="1, Default" w206 {
                tunnel: [w213 w224] -> w207
                tunnel: w208 -> [w212 w223]
                tunnel: [w211 w221] -> w205
                frame 1, Default {
                  # "Ramp ON"
                  n62 = Unbundle By Name(w212) -> ("Ramp voltage ramp rate"=w216:dbl, "Ramp voltage V1 time"=w219:dbl, "Ramp voltatge V2 time"=w220:dbl, "Ramp voltage set point 1(V1)"=w218:dbl, "Ramp voltage set point 2(V2)"=w217:dbl, "Source signal loop count"=w211:i64)
                  n63 = call "Calculate Time to Achieve Slew Rate.vi"("Current/voltage set point 2"=w217, "Current/voltage set point 1"=w218, "Current/voltage slew rate"=w216) -> ("Calculated time"=w215:dbl)  [unwired: 8 in]
                  n64 = Compound Arithmetic op=ADD(w215, w219, w220) -> (w214:dbl)
                  n65 = To Long Integer(number=w214) -> (32bit integer=w213:i32)
                }
                frame 0 {
                  # "Ramp OFF Trap ON"
                  n66 = Unbundle By Name(w223) -> ("Trapezoid voltage falling slew rate"=w230:dbl, "Trapezoid voltage rising slew rate"=w228:dbl, "Trapezoid voltage delay t1"=w233:dbl, "Trapezoid voltage delay t2"=w231:dbl, "Trapezoid voltatge pulse duration"=w232:dbl, "Trapezoid voltage set point 1(V1)"=w226:dbl, "Trapezoid voltage set point 2(V2)"=w225:dbl, "Source signal loop count"=w221:i64)
                  n67 = call "Calculate Time to Achieve Slew Rate.vi"("Current/voltage set point 2"=w226, "Current/voltage set point 1"=w225, "Current/voltage slew rate"=w230) -> ("Calculated time"=w229:dbl)  [unwired: 8 in]
                  n68 = call "Calculate Time to Achieve Slew Rate.vi"("Current/voltage set point 2"=w225, "Current/voltage set point 1"=w226, "Current/voltage slew rate"=w228) -> ("Calculated time"=w227:dbl)  [unwired: 8 in]
                  n69 = Compound Arithmetic op=ADD(w229, w227, w233, w231, w232) -> (w222:dbl)
                  n70 = To Long Integer(number=w222) -> (32bit integer=w224:i32)
                }
              }
              n71 = Add(x=w209, y=w207) -> (x+y=w210:i32)
            }
            n72 = Multiply(x=w200, y=w199) -> (x*y=w201:i64)
          }
        }
        n73 = Unbundle By Name(w142) -> ("Scope vertical coupling"=w155:enum32{"AC", "DC"}, "Scope probe attenuation"=w156:dbl, "Scope output channel name"=w154:string, "Scope resource name"=w157:string)
        n74 = call <instrlib>:"niScope Initialize With Options.vi"("resource name"=w157, "error in"=w149) -> ("instrument handle"=w172:refnum<k15>, "error out"=w171:errorcluster)  [unwired: 12 in]
        n75 = call-poly <instrlib>:"niScope Get Channel Name (Poly).vi"("instrument handle"=w172, "index"=w154, "error in"=w171) -> ("instrument handle out"=w160:refnum<k15>, "channel name"=w147:string, "error out"=w159:errorcluster)  [unwired: 10 in]
        n76 = call <instrlib>:"niScope Configure Vertical.vi"("instrument handle"=w160, "probe attenuation"=w156, "vertical coupling"=w155, "channels"=w147, "vertical range"=w152, "vertical offset"=0.0, "error in"=w159) -> ("instrument handle out"=w170:refnum<k15>, "error out"=w169:errorcluster)  [unwired: 7 in]
        n77 = Multiply(x=w135, y=w136) -> (x*y=w134:dbl)
        n78 = call <instrlib>:"niScope Configure Chan Characteristics.vi"("instrument handle"=w170, "channels"=w147, "input impedance"=w153, "maximum input frequency"=-1.0 ("Maximum Input Frequency"), "error in"=w169) -> ("instrument handle out"=w167:refnum<k15>, "error out"=w168:errorcluster)  [unwired: 9 in]
        n79 = To Long Integer(number=w134) -> (32bit integer=w133:i32)
        n80 = call <instrlib>:"niScope Configure Horizontal Timing.vi"("instrument handle"=w167, "min sample rate"=w135, "reference position"=0.0 ("Reference Position"), "error in"=w168, "min record length"=w133) -> ("instrument handle out"=w164:refnum<k15>, "error out"=w163:errorcluster)  [unwired: 9 in]
        n81 = Unbundle By Name(w146) -> ("Measure load and scope terminal name"=w145:string)
        n82 = property on="Property Node" class="niScope"(reference=w164, error in=w163, "Trigger Modifier"=w161) -> (reference out=w150:refnum<k15>, error out=w162:errorcluster)
        n83 = call-poly <instrlib>:"niScope Configure Trigger (poly).vi"("instrument handle"=w150, "trigger slope"=w158, "trigger source"=w145, "error in"=w162) -> ("instrument handle out"=w148:refnum<k15>, "error out"=w144:errorcluster)  [unwired: 10 in]
        n84 = Bundle By Name(cluster=w146, "Scope channel name"=w147, "Scope out"=w148, "Measure record length scope"=w133) -> (w173:T3)
      }
      frame "ConfigureSourceToSequence" {
        w270 = T7 1028 items=["Seconds"=1028, "Powerline Cycles"=1029] ("aperture time units")
        w277 = 1027 items=["Automatically after Source Complete"=1025, "On Demand"=1026, "On Measure Trigger"=1027] ("Measurement:Advanced:Measure When")
        w282 = 1 items=["Off", "On"] ("DC Voltage:Voltage Level Autorange")
        w281 = T8 1006 items=["DC Voltage"=1006, "DC Current"=1007, "Pulse Voltage"=1049, "Pulse Current"=1050] ("output function")
        w280 = T5 1021 items=["Single Point"=1020, "Sequence"=1021] ("source mode")
        n85 = Unbundle By Name(w248) -> ("Source sample rate"=w260:dbl, "Source transient response"=w255:i32, "Source voltage gain bandwidth"=w269:dbl, "Source voltage compensation frequency"=w268:dbl, "Source voltage pole-zero ratio"=w267:dbl, "Source sample rate"=w238:dbl, "Source signal loop count"=w234:i64, "Source signal logging"=w242:u32[], "Ramp signal enable/disable"=w246:bool, "Trapezoid signal enable/disable"=w245:bool)
        n86 = Unbundle By Name(w259) -> ("Source channel name"=w250:string, "Source out"=w258:refnum<k15>, "Start source terminal name"=w256:string)
        n87 = Build Array(w246, w245) -> (w247:bool[])
        n88 = Boolean Array To Number(Boolean array=w247) -> (number=w244:u32)
        n89 = case shown="3" w244 {
          tunnel: [w289 w320 w351] -> w237
          tunnel: [w288 w316 w353] -> w241
          tunnel: [w287 w315 w352] -> w240
          tunnel: w248 -> [w292 w319 w357]
          tunnel: w242 -> [_ _ w356]
          tunnel: w234 -> [w286 w314 w350]
          frame 1, Default {
            # "Ramp ON Trap OFF"
            n90 = for {
              N: w286 -> [_]
              tunnel: w292 -> [w302]
              shift-right: [w296] -> w288
              shift-left: dbl[] [] -> [w299]
              shift-right: [w295] -> w287
              shift-left: dbl[] [] -> [w298]
              tunnel: [w301] -> w289
              tunnel: w286 -> [w293]
              n91 = Unbundle By Name(w302) -> ("Ramp voltage ramp rate"=w304:dbl, "Ramp voltage V1 time"=w310:dbl, "Ramp voltatge V2 time"=w313:dbl, "Ramp voltage set point 1(V1)"=w309:dbl, "Ramp voltage set point 2(V2)"=w308:dbl, "Ramp voltage V1 time"=w312:dbl, "Ramp voltatge V2 time"=w311:dbl, "Ramp voltage ramp rate"=w307:dbl)
              n92 = call "Calculate Time to Achieve Slew Rate.vi"("Current/voltage set point 2"=w308, "Current/voltage set point 1"=w309, "Current/voltage slew rate"=w304) -> ("Calculated time"=w303:dbl)  [unwired: 8 in]
              n93 = call "Calculate Current or Voltage Values from Slew Rate.vi"("Current/voltage slew rate"=w307, "Current/voltage end point"=w308, "Current/voltage start point"=w309) -> ("Source delays"=w305:dbl[], "Current/voltage values"=w306:dbl[])  [unwired: 7 in]
              n94 = Build Array (concatenate)(w309, w306, w308) -> (w294:dbl[])
              n95 = Build Array (concatenate)(w312, w305, w311) -> (w297:dbl[])
              n96 = Compound Arithmetic op=ADD(w303, w310, w313) -> (w300:dbl)
              n97 = Build Array (concatenate)(w297, w298) -> (w295:dbl[])
              n98 = Build Array (concatenate)(w299, w294) -> (w296:dbl[])
              n99 = Multiply(x=w293, y=w300) -> (x*y=w301:dbl)
            }
          }
          frame 2 {
            # "Ramp OFF Trap ON"
            n100 = for {
              N: w314 -> [_]
              tunnel: [w322] -> w320
              tunnel: w319 -> [w330]
              shift-right: [w323] -> w315
              shift-left: dbl[] [] -> [w327]
              shift-right: [w324] -> w316
              shift-left: dbl[] [] -> [w326]
              tunnel: w314 -> [w321]
              n101 = Unbundle By Name(w330) -> ("Trapezoid voltage falling slew rate"=w343:dbl, "Trapezoid voltage rising slew rate"=w341:dbl, "Trapezoid voltage delay t1"=w349:dbl, "Trapezoid voltage delay t2"=w344:dbl, "Trapezoid voltatge pulse duration"=w348:dbl, "Trapezoid voltage set point 1(V1)"=w339:dbl, "Trapezoid voltage set point 2(V2)"=w335:dbl, "Trapezoid voltage set point 1(V1)"=w334:dbl, "Trapezoid voltage delay t1"=w347:dbl, "Trapezoid voltatge pulse duration"=w346:dbl, "Trapezoid voltage delay t2"=w345:dbl, "Trapezoid voltage rising slew rate"=w338:dbl, "Trapezoid voltage falling slew rate"=w333:dbl)
              n102 = call "Calculate Time to Achieve Slew Rate.vi"("Current/voltage set point 2"=w339, "Current/voltage set point 1"=w335, "Current/voltage slew rate"=w343) -> ("Calculated time"=w342:dbl)  [unwired: 8 in]
              n103 = call "Calculate Time to Achieve Slew Rate.vi"("Current/voltage set point 2"=w335, "Current/voltage set point 1"=w339, "Current/voltage slew rate"=w341) -> ("Calculated time"=w340:dbl)  [unwired: 8 in]
              n104 = call "Calculate Current or Voltage Values from Slew Rate.vi"("Current/voltage slew rate"=w338, "Current/voltage end point"=w335, "Current/voltage start point"=w339) -> ("Source delays"=w336:dbl[], "Current/voltage values"=w337:dbl[])  [unwired: 7 in]
              n105 = call "Calculate Current or Voltage Values from Slew Rate.vi"("Current/voltage slew rate"=w333, "Current/voltage end point"=w334, "Current/voltage start point"=w335) -> ("Source delays"=w331:dbl[], "Current/voltage values"=w332:dbl[])  [unwired: 7 in]
              n106 = Build Array (concatenate)(w339, w337, w335, w332, w334) -> (w325:dbl[])
              n107 = Build Array (concatenate)(w347, w336, w346, w331, w345) -> (w328:dbl[])
              n108 = Compound Arithmetic op=ADD(w342, w340, w349, w344, w348) -> (w329:dbl)
              n109 = Build Array (concatenate)(w326, w325) -> (w324:dbl[])
              n110 = Build Array (concatenate)(w328, w327) -> (w323:dbl[])
              n111 = Multiply(x=w321, y=w329) -> (x*y=w322:dbl)
            }
          }
          frame 3 {
            # "Ramp ON Trap ON"
            n112 = for {
              N: w350 -> [_]
              tunnel: w357 -> [w368]
              tunnel: w356 -> [w367]
              shift-right: [w361] -> w353
              shift-left: dbl[] [] -> [w362]
              shift-right: [w364] -> w352
              shift-left: dbl[] [] -> [w365]
              tunnel: [w359] -> w351
              tunnel: w350 -> [w358]
              n113 = for {
                tunnel: w367 -> [w382] mode=indexing
                shift-right: [w381] -> w363
                shift-left: dbl[] [] -> [w379]
                shift-right: [w377] -> w366
                shift-left: dbl[] [] -> [w376]
                shift-right: [w375] -> w360
                shift-left: 0 -> [w374]
                tunnel: w368 -> [w372]
                n114 = case shown="0" w382 {
                  tunnel: [w385 w398] -> w373
                  tunnel: [w386 w401] -> w380
                  tunnel: [w384 w400] -> w378
                  tunnel: w372 -> [w383 w399]
                  frame 1, Default {
                    # "Ramp ON"
                    n115 = Unbundle By Name(w383) -> ("Ramp voltage ramp rate"=w388:dbl, "Ramp voltage V1 time"=w394:dbl, "Ramp voltatge V2 time"=w397:dbl, "Ramp voltage set point 1(V1)"=w393:dbl, "Ramp voltage set point 2(V2)"=w392:dbl, "Ramp voltage V1 time"=w396:dbl, "Ramp voltatge V2 time"=w395:dbl, "Ramp voltage ramp rate"=w391:dbl)
                    n116 = call "Calculate Time to Achieve Slew Rate.vi"("Current/voltage set point 2"=w392, "Current/voltage set point 1"=w393, "Current/voltage slew rate"=w388) -> ("Calculated time"=w387:dbl)  [unwired: 8 in]
                    n117 = call "Calculate Current or Voltage Values from Slew Rate.vi"("Current/voltage slew rate"=w391, "Current/voltage end point"=w392, "Current/voltage start point"=w393) -> ("Source delays"=w389:dbl[], "Current/voltage values"=w390:dbl[])  [unwired: 7 in]
                    n118 = Build Array (concatenate)(w393, w390, w392) -> (w386:dbl[])
                    n119 = Build Array (concatenate)(w396, w389, w395) -> (w384:dbl[])
                    n120 = Compound Arithmetic op=ADD(w387, w394, w397) -> (w385:dbl)
                  }
                  frame 0 {
                    # "Trap voltage values and time"
                    n121 = Unbundle By Name(w399) -> ("Trapezoid voltage falling slew rate"=w414:dbl, "Trapezoid voltage rising slew rate"=w412:dbl, "Trapezoid voltage delay t1"=w420:dbl, "Trapezoid voltage delay t2"=w415:dbl, "Trapezoid voltatge pulse duration"=w419:dbl, "Trapezoid voltage set point 1(V1)"=w410:dbl, "Trapezoid voltage set point 2(V2)"=w406:dbl, "Trapezoid voltage set point 1(V1)"=w405:dbl, "Trapezoid voltage delay t1"=w418:dbl, "Trapezoid voltatge pulse duration"=w417:dbl, "Trapezoid voltage delay t2"=w416:dbl, "Trapezoid voltage rising slew rate"=w409:dbl, "Trapezoid voltage falling slew rate"=w404:dbl)
                    n122 = call "Calculate Time to Achieve Slew Rate.vi"("Current/voltage set point 2"=w410, "Current/voltage set point 1"=w406, "Current/voltage slew rate"=w414) -> ("Calculated time"=w413:dbl)  [unwired: 8 in]
                    n123 = call "Calculate Time to Achieve Slew Rate.vi"("Current/voltage set point 2"=w406, "Current/voltage set point 1"=w410, "Current/voltage slew rate"=w412) -> ("Calculated time"=w411:dbl)  [unwired: 8 in]
                    n124 = call "Calculate Current or Voltage Values from Slew Rate.vi"("Current/voltage slew rate"=w409, "Current/voltage end point"=w406, "Current/voltage start point"=w410) -> ("Source delays"=w407:dbl[], "Current/voltage values"=w408:dbl[])  [unwired: 7 in]
                    n125 = call "Calculate Current or Voltage Values from Slew Rate.vi"("Current/voltage slew rate"=w404, "Current/voltage end point"=w405, "Current/voltage start point"=w406) -> ("Source delays"=w402:dbl[], "Current/voltage values"=w403:dbl[])  [unwired: 7 in]
                    n126 = Build Array (concatenate)(w410, w408, w406, w403, w405) -> (w401:dbl[])
                    n127 = Build Array (concatenate)(w418, w407, w417, w402, w416) -> (w400:dbl[])
                    n128 = Compound Arithmetic op=ADD(w413, w411, w420, w415, w419) -> (w398:dbl)
                  }
                }
                n129 = Build Array (concatenate)(w379, w380) -> (w381:dbl[])
                n130 = Add(x=w374, y=w373) -> (x+y=w375:dbl)
                n131 = Build Array (concatenate)(w378, w376) -> (w377:dbl[])
              }
              n132 = Build Array (concatenate)(w362, w363) -> (w361:dbl[])
              n133 = Build Array (concatenate)(w366, w365) -> (w364:dbl[])
              n134 = Multiply(x=w358, y=w360) -> (x*y=w359:dbl)
            }
          }
        }
        n135 = call <instrlib>:"niDCPower Configure Source Mode With Channels.vi"("error in (no error)"=w257, "source mode"=w280, "channel name"=w250, "instrument handle"=w258) -> ("error out"=w278:errorcluster, "instrument handle out"=w279:refnum<k15>)  [unwired: 6 in]
        n136 = call <instrlib>:"niDCPower Configure Output Function.vi"("error in (no error)"=w278, "output function"=w281, "channel name"=w250, "instrument handle"=w279) -> ("error out"=w274:errorcluster, "instrument handle out"=w272:refnum<k15>)  [unwired: 6 out]
        n137 = Reciprocal(x=w260) -> (1/x=w243:dbl)
        n138 = call <instrlib>:"niDCPower Configure Aperture Time.vi"("aperture time units"=w270, "error in (no error)"=w274, "aperture time"=w243, "channel name"=w250, "instrument handle"=w272) -> ("error out"=w273:errorcluster, "instrument handle out"=w271:refnum<k15>)  [unwired: 5 in]
        n139 = property class="niDCPower"(reference=w271, error in=w273, "Active Channel"=w250, "Source:DC Voltage:Voltage Level Autorange"=w282, "Source:DC Voltage:Current Limit Autorange"=w282) -> (reference out=w283:refnum<k15>, error out=w284:errorcluster)
        n140 = Multiply(x=w238, y=w237) -> (x*y=w236:dbl)
        n141 = To Long Integer(number=w236) -> (32bit integer=w235:i32)
        n142 = property class="niDCPower"(reference=w283, error in=w284, "Active Channel"=w250, "Measure Record Length"=w235, "Transient Response"=w255, "Voltage GBW"=w269, "Voltage Compensation Freq"=w268, "Voltage Pole-Zero Ratio"=w267) -> (reference out=w265:refnum<k15>, error out=w266:errorcluster)
        n143 = call <instrlib>:"niDCPower Set Sequence.vi"("source delays"=w240, "error in (no error)"=w266, "values"=w241, "channel name"=w250, "instrument handle"=w265) -> ("error out"=w263:errorcluster, "instrument handle out"=w264:refnum<k15>)  [unwired: 5 in]
        n144 = call-poly <instrlib>:"niDCPower Configure Trigger With Channels (Poly).vi"("error in (no error)"=w263, "input terminal"=w256, "channel name"=w250, "instrument handle"=w264) -> ("error out"=w261:errorcluster, "instrument handle out"=w262:refnum<k15>)  [unwired: 6 in]
        n145 = property class="niDCPower"(reference=w262, error in=w261, "Measure When"=w277, "Aperture Time"=w243) -> (reference out=w275:refnum<k15>, error out=w276:errorcluster)
        n146 = call <instrlib>:"niDCPower Commit With Channels.vi"("error in (no error)"=w276, "channel name"=w250, "instrument handle"=w275) -> ("error out"=w253:errorcluster, "instrument handle out"=w252:refnum<k15>)  [unwired: 7 in]
        n147 = property class="niDCPower"(reference=w252, error in=w253, "Active Channel"=w250) -> (reference out=w251:refnum<k15>, error out=w249:errorcluster, "Measure Record dt"=w239:dbl)
        n148 = Bundle By Name(cluster=w259, "Source channel name"=w250, "Source out"=w251, "Measurement Results.Source voltage dt"=w239, "Measure record length smu"=w235, "Measurement Results.Load voltage dt"=w239) -> (w285:T3)
      }
      frame "ConfigureLoadToSinglePoint" {
        w430 = 1027 items=["Automatically after Source Complete"=1025, "On Demand"=1026, "On Measure Trigger"=1027] ("Measurement:Advanced:Measure When")
        w440 = T8 1007 items=["DC Voltage"=1006, "DC Current"=1007, "Pulse Voltage"=1049, "Pulse Current"=1050] ("output function")
        w439 = T5 1020 items=["Single Point"=1020, "Sequence"=1021] ("source mode")
        n149 = Unbundle By Name(w423) -> ("Load channel name"=w425:string, "Load out"=w446:refnum<k15>)
        n150 = Unbundle By Name(w423) -> ("Measure record length smu"=w433:i32, "Aperture time"=w432:dbl)
        n151 = Unbundle By Name(w423) -> ("Source terminal name"=w445:string, "Measure load and scope terminal name"=w444:string)
        n152 = call <instrlib>:"niDCPower Configure Source Mode With Channels.vi"("error in (no error)"=w424, "source mode"=w439, "channel name"=w425, "instrument handle"=w446) -> ("error out"=w437:errorcluster, "instrument handle out"=w438:refnum<k15>)  [unwired: 6 in]
        n153 = call <instrlib>:"niDCPower Configure Output Function.vi"("error in (no error)"=w437, "output function"=w440, "channel name"=w425, "instrument handle"=w438) -> ("error out"=w442:errorcluster, "instrument handle out"=w441:refnum<k15>)  [unwired: 6 out]
        n154 = call-poly <instrlib>:"niDCPower Configure Trigger With Channels (Poly).vi"("error in (no error)"=w442, "input terminal"=w445, "channel name"=w425, "instrument handle"=w441) -> ("error out"=w434:errorcluster, "instrument handle out"=w443:refnum<k15>)  [unwired: 6 in]
        n155 = property class="niDCPower"(reference=w443, error in=w434, "Measure Record Length"=w433, "Aperture Time"=w432) -> (reference out=w436:refnum<k15>, error out=w435:errorcluster)
        n156 = call-poly <instrlib>:"niDCPower Configure Trigger With Channels (Poly).vi"("error in (no error)"=w435, "input terminal"=w444, "channel name"=w425, "instrument handle"=w436) -> ("error out"=w429:errorcluster, "instrument handle out"=w427:refnum<k15>)  [unwired: 6 in]
        n157 = property class="niDCPower"(reference=w427, error in=w429, "Measure When"=w430) -> (reference out=w426:refnum<k15>, error out=w428:errorcluster)
        n158 = call <instrlib>:"niDCPower Commit With Channels.vi"("error in (no error)"=w428, "channel name"=w425, "instrument handle"=w426) -> ("error out"=w421:errorcluster, "instrument handle out"=w431:refnum<k15>)  [unwired: 7 in]
        n159 = Bundle By Name(cluster=w423, "Load out"=w431) -> (w422:T3)
      }
      frame "StartSource" {
        n160 = Unbundle By Name(w452) -> ("Source out"=w448:refnum<k15>, "Source channel name"=w454:string)
        n161 = flat-sequence {
          tunnel: [w463] -> w458
          tunnel: [w462] -> w457
          tunnel: w448 -> [w461]
          tunnel: w454 -> [w459]
          tunnel: [w459] -> w456
          tunnel: w453 -> [w460]
          tunnel: w458 -> [w468]
          tunnel: w457 -> [w467]
          tunnel: [w465] -> w455
          tunnel: [w466] -> w450
          tunnel: w456 -> [w464]
          frame #0 {
            n162 = call <instrlib>:"niDCPower Initiate With Channels.vi"("error in (no error)"=w460, "channel name"=w459, "instrument handle"=w461) -> ("error out"=w462:errorcluster, "instrument handle out"=w463:refnum<k15>)  [unwired: 7 in]
          }
          frame #1 {
            w469 = T4 1033 items=["Source Complete Event"=1030, "Measure Complete Event"=1031, "Sequence Iteration Complete Event"=1032, "Sequence Engine Done Event"=1033] ("event")
            n163 = call <instrlib>:"niDCPower Wait For Event With Channels.vi"("error in (no error)"=w467, "event"=w469, "channel name"=w464, "instrument handle"=w468) -> ("error out"=w466:errorcluster, "instrument handle out"=w465:refnum<k15>)  [unwired: 6 in]
          }
        }
        n164 = Bundle By Name(cluster=w452, "Source out"=w455) -> (w451:T3)
      }
      frame "StartSourceandLoad" {
        n165 = Unbundle By Name(w472) -> ("Source out"=w474:refnum<k15>, "Source channel name"=w475:string, "Load out"=w478:refnum<k15>, "Load channel name"=w479:string)
        n166 = flat-sequence {
          tunnel: [w492] -> w483
          tunnel: [w491] -> w482
          tunnel: [w490] -> w481
          tunnel: w478 -> [w489]
          tunnel: w474 -> [w488]
          tunnel: w475 -> [w485]
          tunnel: w479 -> [w486]
          tunnel: [w485] -> w480
          tunnel: w473 -> [w487]
          tunnel: w483 -> [w499]
          tunnel: w482 -> [w498]
          tunnel: w481 -> [w495]
          tunnel: [w496] -> w476
          tunnel: [w497] -> w470
          tunnel: [w495] -> w477
          tunnel: w480 -> [w494]
          frame #0 {
            n167 = call <instrlib>:"niDCPower Initiate With Channels.vi"("error in (no error)"=w487, "channel name"=w486, "instrument handle"=w489) -> ("error out"=w493:errorcluster, "instrument handle out"=w490:refnum<k15>)  [unwired: 7 in]
            n168 = call <instrlib>:"niDCPower Initiate With Channels.vi"("error in (no error)"=w493, "channel name"=w485, "instrument handle"=w488) -> ("error out"=w491:errorcluster, "instrument handle out"=w492:refnum<k15>)  [unwired: 7 in]
          }
          frame #1 {
            w500 = T4 1033 items=["Source Complete Event"=1030, "Measure Complete Event"=1031, "Sequence Iteration Complete Event"=1032, "Sequence Engine Done Event"=1033] ("event")
            n169 = call <instrlib>:"niDCPower Wait For Event With Channels.vi"("error in (no error)"=w498, "event"=w500, "channel name"=w494, "instrument handle"=w499) -> ("error out"=w497:errorcluster, "instrument handle out"=w496:refnum<k15>)  [unwired: 6 in]
          }
        }
        n170 = Bundle By Name(cluster=w472, "Source out"=w476, "Load out"=w477) -> (w471:T3)
      }
      frame "StartSourceAndScope" {
        n171 = Unbundle By Name(w508) -> ("Source out"=w511:refnum<k15>, "Source channel name"=w510:string, "Scope out"=w506:refnum<k15>)
        n172 = flat-sequence {
          tunnel: [w522] -> w514
          tunnel: [w515] -> w513
          tunnel: w511 -> [w521]
          tunnel: w510 -> [w516]
          tunnel: [w516] -> w512
          tunnel: w507 -> [w520]
          tunnel: w506 -> [w518]
          tunnel: [w517] -> w505
          tunnel: w514 -> [w528]
          tunnel: w513 -> [w527]
          tunnel: [w525] -> w509
          tunnel: [w526] -> w504
          tunnel: w512 -> [w524]
          tunnel: [w523] -> w501
          tunnel: w505 -> [w523]
          frame #0 {
            n173 = call <instrlib>:"niScope Initiate Acquisition.vi"("instrument handle"=w518, "error in"=w520) -> ("instrument handle out"=w517:refnum<k15>, "error out"=w519:errorcluster)  [unwired: 12 in]
            n174 = call <instrlib>:"niDCPower Initiate With Channels.vi"("error in (no error)"=w519, "channel name"=w516, "instrument handle"=w521) -> ("error out"=w515:errorcluster, "instrument handle out"=w522:refnum<k15>)  [unwired: 7 in]
          }
          frame #1 {
            w529 = T4 1033 items=["Source Complete Event"=1030, "Measure Complete Event"=1031, "Sequence Iteration Complete Event"=1032, "Sequence Engine Done Event"=1033] ("event")
            n175 = call <instrlib>:"niDCPower Wait For Event With Channels.vi"("error in (no error)"=w527, "event"=w529, "channel name"=w524, "instrument handle"=w528) -> ("error out"=w526:errorcluster, "instrument handle out"=w525:refnum<k15>)  [unwired: 6 in]
          }
        }
        n176 = Bundle By Name(cluster=w508, "Source out"=w509, "Scope out"=w501) -> (w503:T3)
      }
      frame "StartSourceLoadAndScope" {
        n177 = Unbundle By Name(w532) -> ("Source out"=w541:refnum<k15>, "Source channel name"=w540:string, "Load out"=w535:refnum<k15>, "Load channel name"=w534:string, "Scope out"=w537:refnum<k15>)
        n178 = flat-sequence {
          tunnel: [w558] -> w546
          tunnel: [w557] -> w545
          tunnel: [w556] -> w544
          tunnel: w535 -> [w555]
          tunnel: w541 -> [w554]
          tunnel: w540 -> [w548]
          tunnel: w534 -> [w549]
          tunnel: [w548] -> w543
          tunnel: w533 -> [w553]
          tunnel: w537 -> [w551]
          tunnel: [w550] -> w542
          tunnel: w546 -> [w566]
          tunnel: w545 -> [w565]
          tunnel: w544 -> [w563]
          tunnel: [w560] -> w539
          tunnel: [w564] -> w530
          tunnel: [w563] -> w538
          tunnel: w543 -> [w562]
          tunnel: [w561] -> w536
          tunnel: w542 -> [w561]
          frame #0 {
            n179 = call <instrlib>:"niScope Initiate Acquisition.vi"("instrument handle"=w551, "error in"=w553) -> ("instrument handle out"=w550:refnum<k15>, "error out"=w552:errorcluster)  [unwired: 12 in]
            n180 = call <instrlib>:"niDCPower Initiate With Channels.vi"("error in (no error)"=w552, "channel name"=w549, "instrument handle"=w555) -> ("error out"=w559:errorcluster, "instrument handle out"=w556:refnum<k15>)  [unwired: 7 in]
            n181 = call <instrlib>:"niDCPower Initiate With Channels.vi"("error in (no error)"=w559, "channel name"=w548, "instrument handle"=w554) -> ("error out"=w557:errorcluster, "instrument handle out"=w558:refnum<k15>)  [unwired: 7 in]
          }
          frame #1 {
            w567 = T4 1033 items=["Source Complete Event"=1030, "Measure Complete Event"=1031, "Sequence Iteration Complete Event"=1032, "Sequence Engine Done Event"=1033] ("event")
            n182 = call <instrlib>:"niDCPower Wait For Event With Channels.vi"("error in (no error)"=w565, "event"=w567, "channel name"=w562, "instrument handle"=w566) -> ("error out"=w564:errorcluster, "instrument handle out"=w560:refnum<k15>)  [unwired: 6 in]
          }
        }
        n183 = Bundle By Name(cluster=w532, "Source out"=w539, "Load out"=w538, "Scope out"=w536) -> (w531:T3)
      }
      frame "PerformMeasurement" {
        n184 = Unbundle By Name(w573) -> ("Load enable/disable"=w572:bool, "Scope enable/disable"=w580:bool)
        n185 = Unbundle By Name(w592) -> ("Source out"=w589:refnum<k15>, "Source channel name"=w588:string, "Measure record length smu"=w576:i32, "Load out"=w578:refnum<k15>, "Load channel name"=w577:string)
        n186 = Unbundle By Name(w592) -> ("Scope out"=w587:refnum<k15>, "Scope channel name"=w586:string, "Measure record length scope"=w584:i32)
        n187 = call <instrlib>:"niDCPower Fetch Multiple.vi"("instrument handle"=w589, "channel name"=w588, "count (1)"=w576, "error in (no error)"=w593) -> ("instrument handle out"=w585:refnum<k15>, "voltage measurements"=w571:dbl[], "error out"=w581:errorcluster)  [unwired: 1 in, 8 out]
        n188 = case shown="False" w572 {
          tunnel: w581 -> [w595 w602]
          tunnel: [w595 w601] -> w579
          tunnel: w578 -> [w594 w600]
          tunnel: w577 -> [_ w599]
          tunnel: w576 -> [_ w598]
          tunnel: [w594 w597] -> w575
          tunnel: [_ w596] -> w570
          frame False {
          }
          frame True {
            n189 = call <instrlib>:"niDCPower Fetch Multiple.vi"("instrument handle"=w600, "channel name"=w599, "count (1)"=w598, "error in (no error)"=w602) -> ("instrument handle out"=w597:refnum<k15>, "voltage measurements"=w596:dbl[], "error out"=w601:errorcluster)  [unwired: 1 in, 8 out]
          }
        }
        n190 = case shown="False" w580 {
          tunnel: [w604 w611] -> w590
          tunnel: w579 -> [w604 w610]
          tunnel: w587 -> [w603 w609]
          tunnel: w586 -> [_ w608]
          tunnel: [w603 w607] -> w574
          tunnel: w584 -> [_ w606]
          tunnel: [_ w605] -> w583
          frame False {
          }
          frame True {
            n191 = call-poly <instrlib>:"niScope Fetch (poly).vi"("error in"=w610, "numSamples"=w606, "channels"=w608, "instrument handle"=w609) -> ("error out"=w611:errorcluster, "wfm"=w605:waveform(dbl), "instrument handle out"=w607:refnum<k15>)  [unwired: 4 in, 1 out]
          }
        }
        n192 = Unbundle By Name(w583) -> ("Y"=w569:dbl[], "dt"=w568:dbl)
        n193 = Bundle By Name(cluster=w592, "Source out"=w585, "Measurement Results.Source voltages"=w571, "Load out"=w575, "Measurement Results.Load voltages"=w570, "Scope out"=w574, "Measurement Results.Scope amplitudes"=w569, "Measurement Results.Scope amplitude dt"=w568) -> (w591:T3)
      }
      frame "Exit", Default {
        n194 = Unbundle By Name(w624) -> ("Scope enable/disable"=w619:bool, "Load enable/disable"=w612:bool)
        n195 = Unbundle By Name(w625) -> ("Source out"=w620:refnum<k15>, "Source channel name"=w621:string, "Load out"=w614:refnum<k15>, "Load channel name"=w613:string, "Scope out"=w615:refnum<k15>)
        n196 = case shown="True" w619 {
          tunnel: w628 -> [w636 w639]
          tunnel: [w636 w638] -> w617
          tunnel: w615 -> [_ w637]
          frame False {
          }
          frame True {
            n197 = call <instrlib>:"niScope Close.vi"("instrument handle"=w637, "error in"=w639) -> ("error out"=w638:errorcluster)  [unwired: 13 in]
          }
        }
        n198 = case shown="True" w612 {
          tunnel: w617 -> [w629 w633]
          tunnel: [w629 w632] -> w616
          tunnel: w614 -> [_ w631]
          tunnel: w613 -> [_ w630]
          frame False {
          }
          frame True {
            n199 = call <instrlib>:"niDCPower Abort With Channels.vi"("error in (no error)"=w633, "channel name"=w630, "instrument handle"=w631) -> ("error out"=w635:errorcluster, "instrument handle out"=w634:refnum<k15>)  [unwired: 7 in]
            n200 = call <instrlib>:"niDCPower Close.vi"("error in (no error)"=w635, "instrument handle"=w634) -> ("error out"=w632:errorcluster)  [unwired: 9 in]
          }
        }
        n201 = call <instrlib>:"niDCPower Abort With Channels.vi"("error in (no error)"=w616, "channel name"=w621, "instrument handle"=w620) -> ("error out"=w623:errorcluster, "instrument handle out"=w622:refnum<k15>)  [unwired: 7 in]
        n202 = call <instrlib>:"niDCPower Close.vi"("error in (no error)"=w623, "instrument handle"=w622) -> ("error out"=w627:errorcluster)  [unwired: 9 in]
      }
    }
  }
  "error out" <- w5
  "measure call context out" <- w6
  n203 = Unbundle By Name(w3) -> ("Measurement Results"=→"measurement results":T2)
